vi "3D Experiment Final kinect.vi"() -> ()   [LabVIEW 2011]
uses:
  <vilib>/Platform/TimedLoop/XDataNode/timing_clust.ctl
  <vilib>/Platform/TimedLoop/XDataNode/nitl_modes.ctl
  <vilib>/Platform/TimedLoop/XDataNode/wakeup.ctl
  <vilib>/Utility/miscctls.llb/LV3DPointTypeDef.ctl
  <vilib>/Utility/miscctls.llb/LVRGBAColorTypeDef.ctl
  <vilib>/Utility/cursorutil.llb/Set Cursor (Cursor ID).vi
  <vilib>/Utility/inputDevices.llb/closeMouse.vi
  <vilib>/Utility/inputDevices.llb/mouseAcquire.vi
  <vilib>/Utility/file.llb/Write To Spreadsheet File (DBL).vi
  <vilib>/Utility/file.llb/Write To Spreadsheet File (I64).vi
  <vilib>/Platform/TimedLoop/XDataNode/XDataNode.xnode
  <vilib>/picture/3D Picture Control/NI_3D Picture Control.lvlib
  <vilib>/Platform/TimedLoop/XDataNode/XDNodeRunTimeDep.lvlib
  kinect-1-4/Kinect_API.lvlib
panel:
  in  "Far object filter 2":i32(slide)=26869 scale=0.0..4305.0
  out "click 2":bool
  out "stop":bool
  in  "Replace with?":i32=60000
  out "initial time 2":u32
  out "initial time":u32
  in  "stop":bool
  out "3D Picture":refnum<vi>(3d-picture)
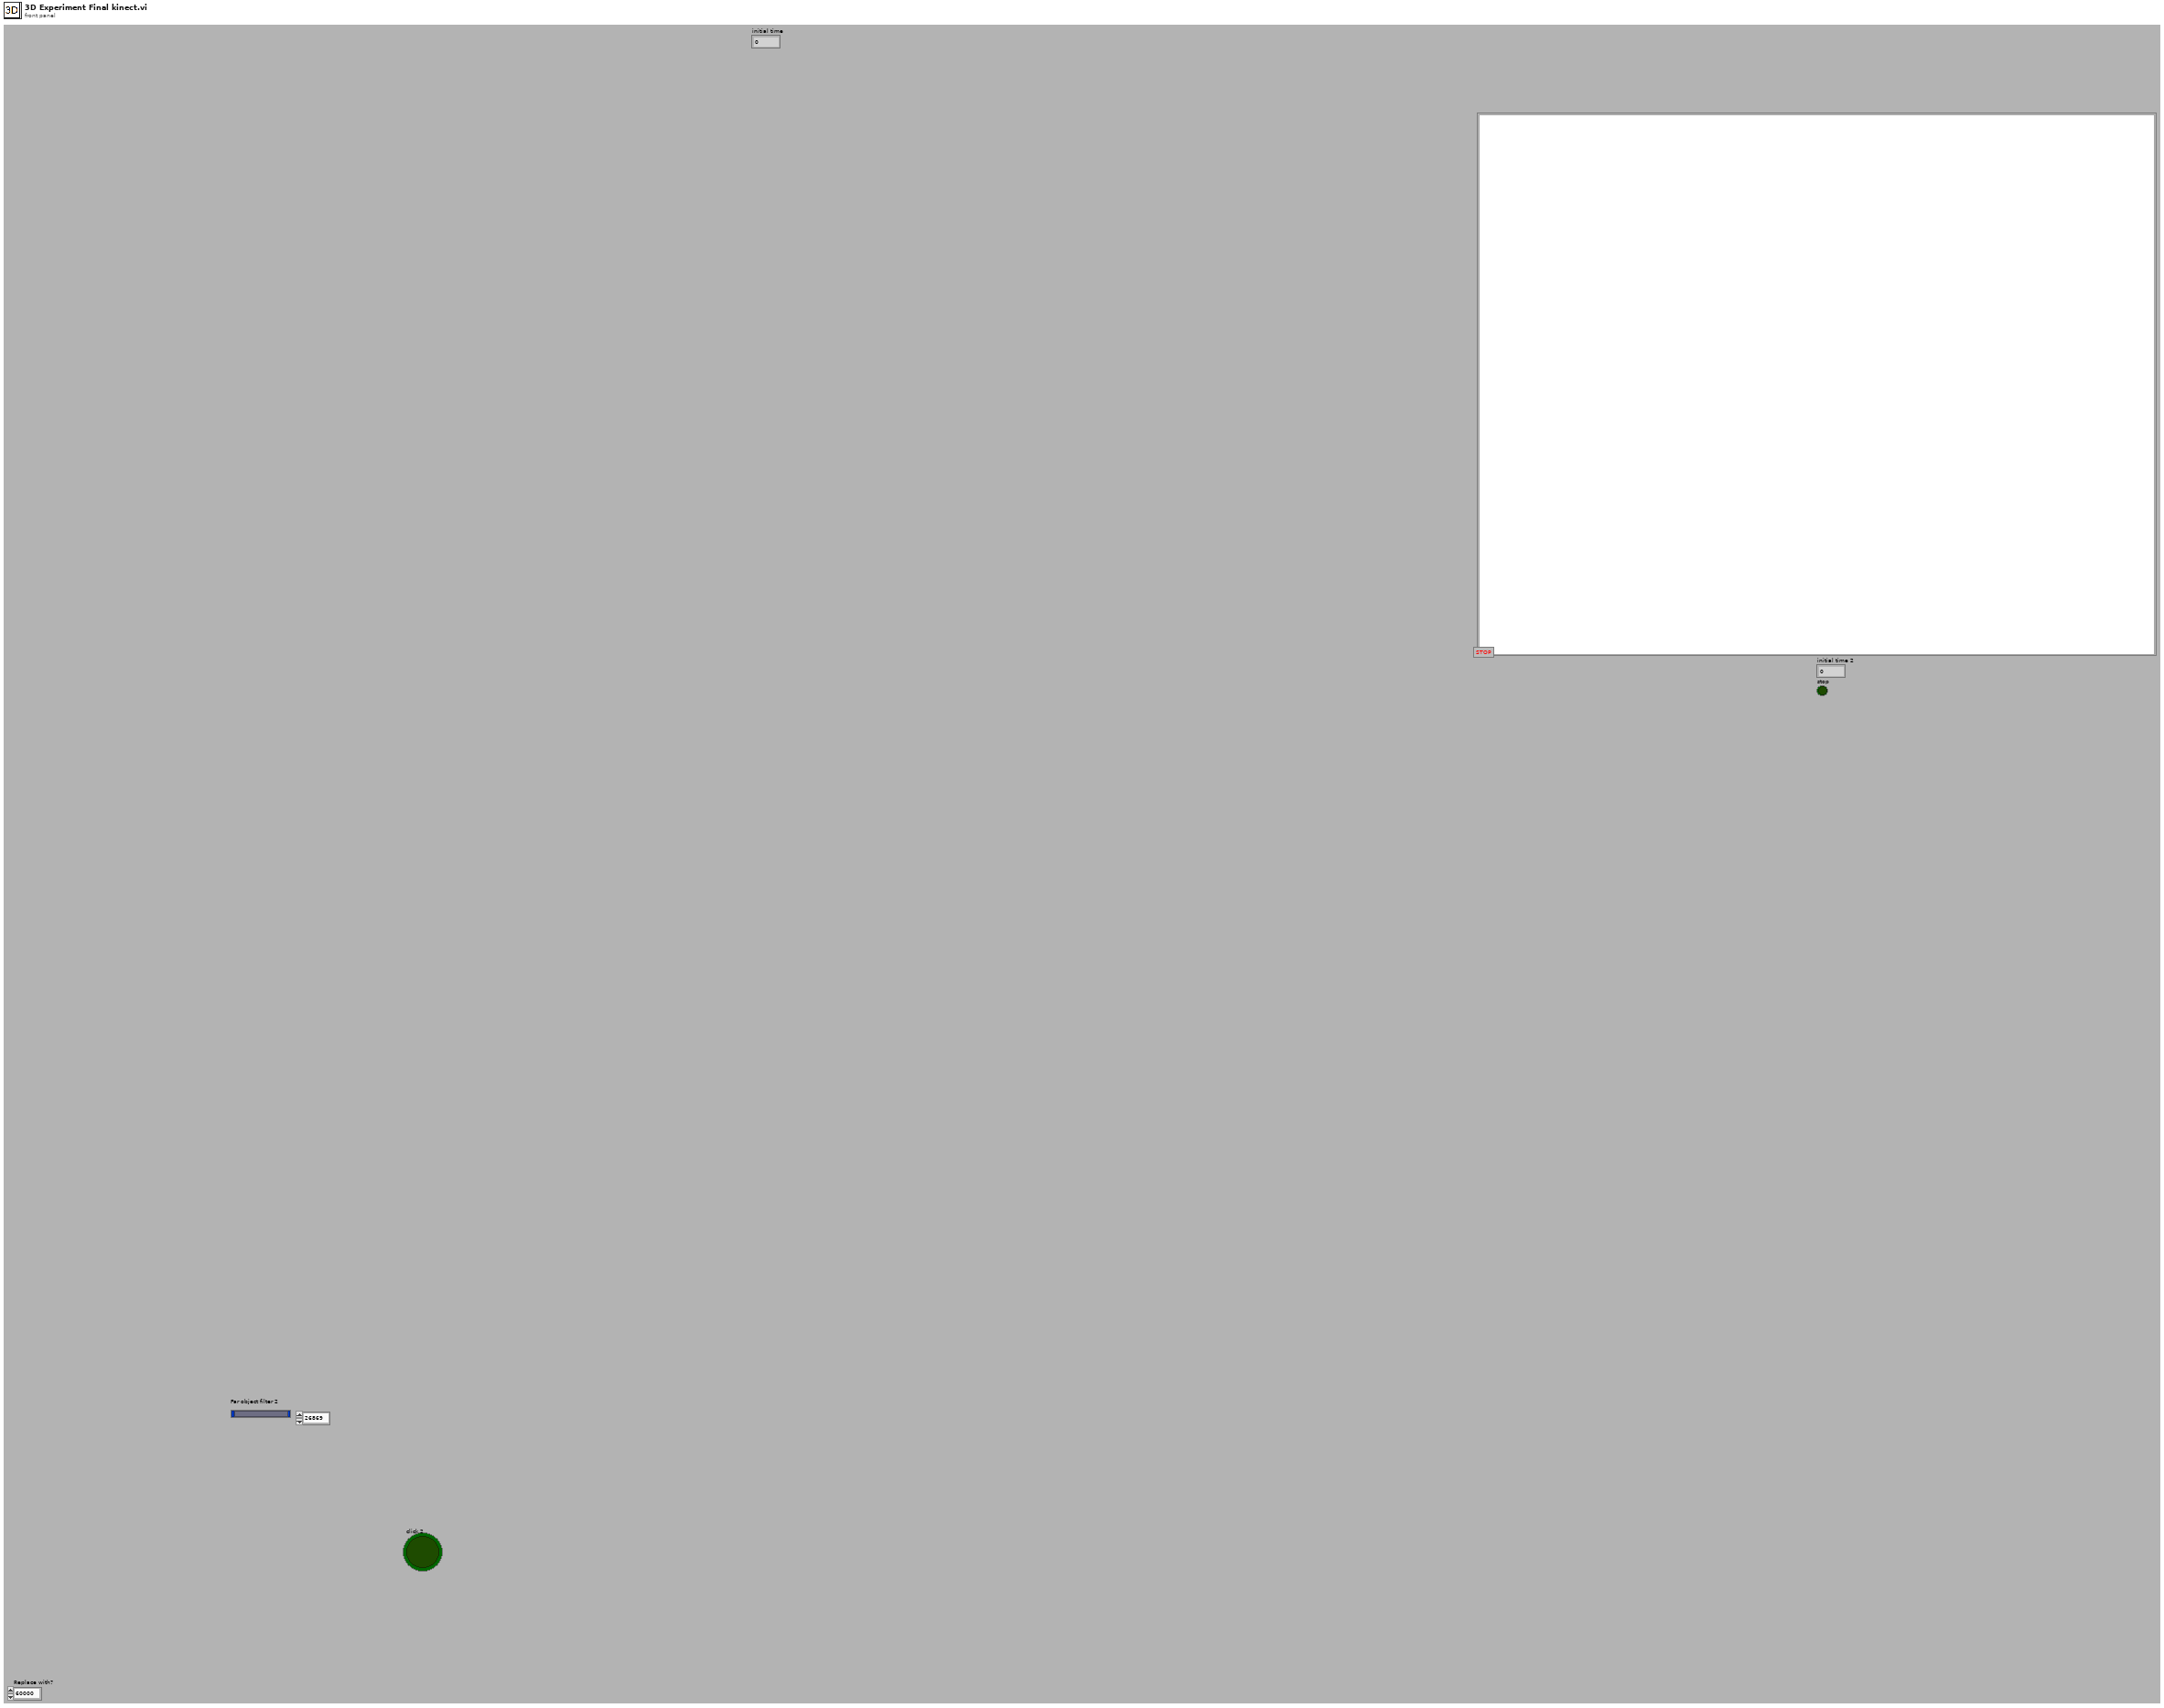
[diagram p1: front panel]
types:
  T1 = enum16{"open", "replace", "create", "open or create", "replace or create", "replace or create with confirmation"}
  T2 = typedef "LV3DPointTypeDef.ctl" = cluster{"X":sgl, "Y":sgl, "Z":sgl}
  T3 = enum16{"Inherit Value", "Points", "Wireframe", "Polygons"}
  T4 = enum16{"Inherit Value", "No Culling", "Cull Back Face", "Cull Front Face", "Cull Both Faces"}
  T5 = enum16{"Zero", "One", "Destination Color", "One Minus Destination Color", "Source Alpha", "One Minus Source Alpha", "Destination Alpha", "One Minus Destination Alpha", "Source Alpha Saturate"}
  T6 = enum16{"Zero", "One", "Source Color", "One Minus Source Color", "Source Alpha", "One Minus Source Alpha", "Destination Alpha", "One Minus Destination Alpha"}
  T7 = enum16{"Normal Bin", "Opaque Bin", "Transparent Bin"}
  T8 = typedef "XDNodeRunTimeDep.lvlib/timing_clust.ctl" = cluster{"Expected End [f-1]":u64, "Actual End [f-1]":u64, "Finished Late? [f-1]":bool, "Expected End [i-1]":u64, "Actual End [i-1]":u64, "Finished Late? [i-1]":bool, "Expected Start [i]":u64, "Actual Start [i]":u64, "Expected Start [f]":u64, "Actual Start [f]":u64, "Source Name":string, "Structure Name":string, "Period":i64, "Deadline":i64, "Offset":i64, "Start":i64, "Priority":i32, "Timeout":i32, "Mode":T9, "Wakeup Reason":T10, "Error":errorcluster, "Source Type":string, "Secondary Source Type":string, "Global End Time":u64, "Global Start Time":u64, "Frame Duration":u64, "Iteration Duration":u64, "Assigned CPU":i32, "I/O Scan Engine Mode":u32}
  T9 = typedef "XDNodeRunTimeDep.lvlib/nitl_modes.ctl" = enum32{"No Change", "Process missed periods, maintain original phase", "Discard missed periods, maintain original phase", "Process missed periods, ignore original phase", "Discard missed periods, ignore original phase"}
  T10 = typedef "XDNodeRunTimeDep.lvlib/wakeup.ctl" = enum32{"Normal", "Aborted", "Asynchronous wakeup", "Timing source error", "Timed loop error", "Timeout"}
  T11 = cluster{"Red":sgl, "Green":sgl, "Blue":sgl, "Alpha":sgl}
  T12 = typedef "LVRGBAColorTypeDef.ctl" = cluster{"Red":sgl, "Green":sgl, "Blue":sgl, "Alpha":sgl}
  T13 = typedef "LVAllMonitorsDisplayTypeDef.ctl" = cluster{"Bounds":cluster{"Left":i16, "Top":i16, "Right":i16, "Bottom":i16}, "Depth":i16}[]
  T14 = cluster{"Bounds":cluster{"Left":i16, "Top":i16, "Right":i16, "Bottom":i16}, "Depth":i16}
  T15 = cluster{"Left":i16, "Top":i16, "Right":i16, "Bottom":i16}
  T16 = cluster{"element":dbl, "Y_scaling":dbl, "element":dbl}
  T17 = cluster{"queue out":refnum<queue>, "queue out":refnum<queue>}
  T18 = cluster{"new reference":refnum<k24>, "DepthStream":refnum<k24>, "VideoStream":refnum<k24>, "Event Callback":refnum<k27>, "Event Callback":refnum<k27>}
  T19 = cluster{"button 1":bool, "button 2":bool, "button 3":bool, "button 4":bool}
  T20 = cluster{"\naverage Y":dbl, "\naverage X ":dbl, "average Z":dbl}
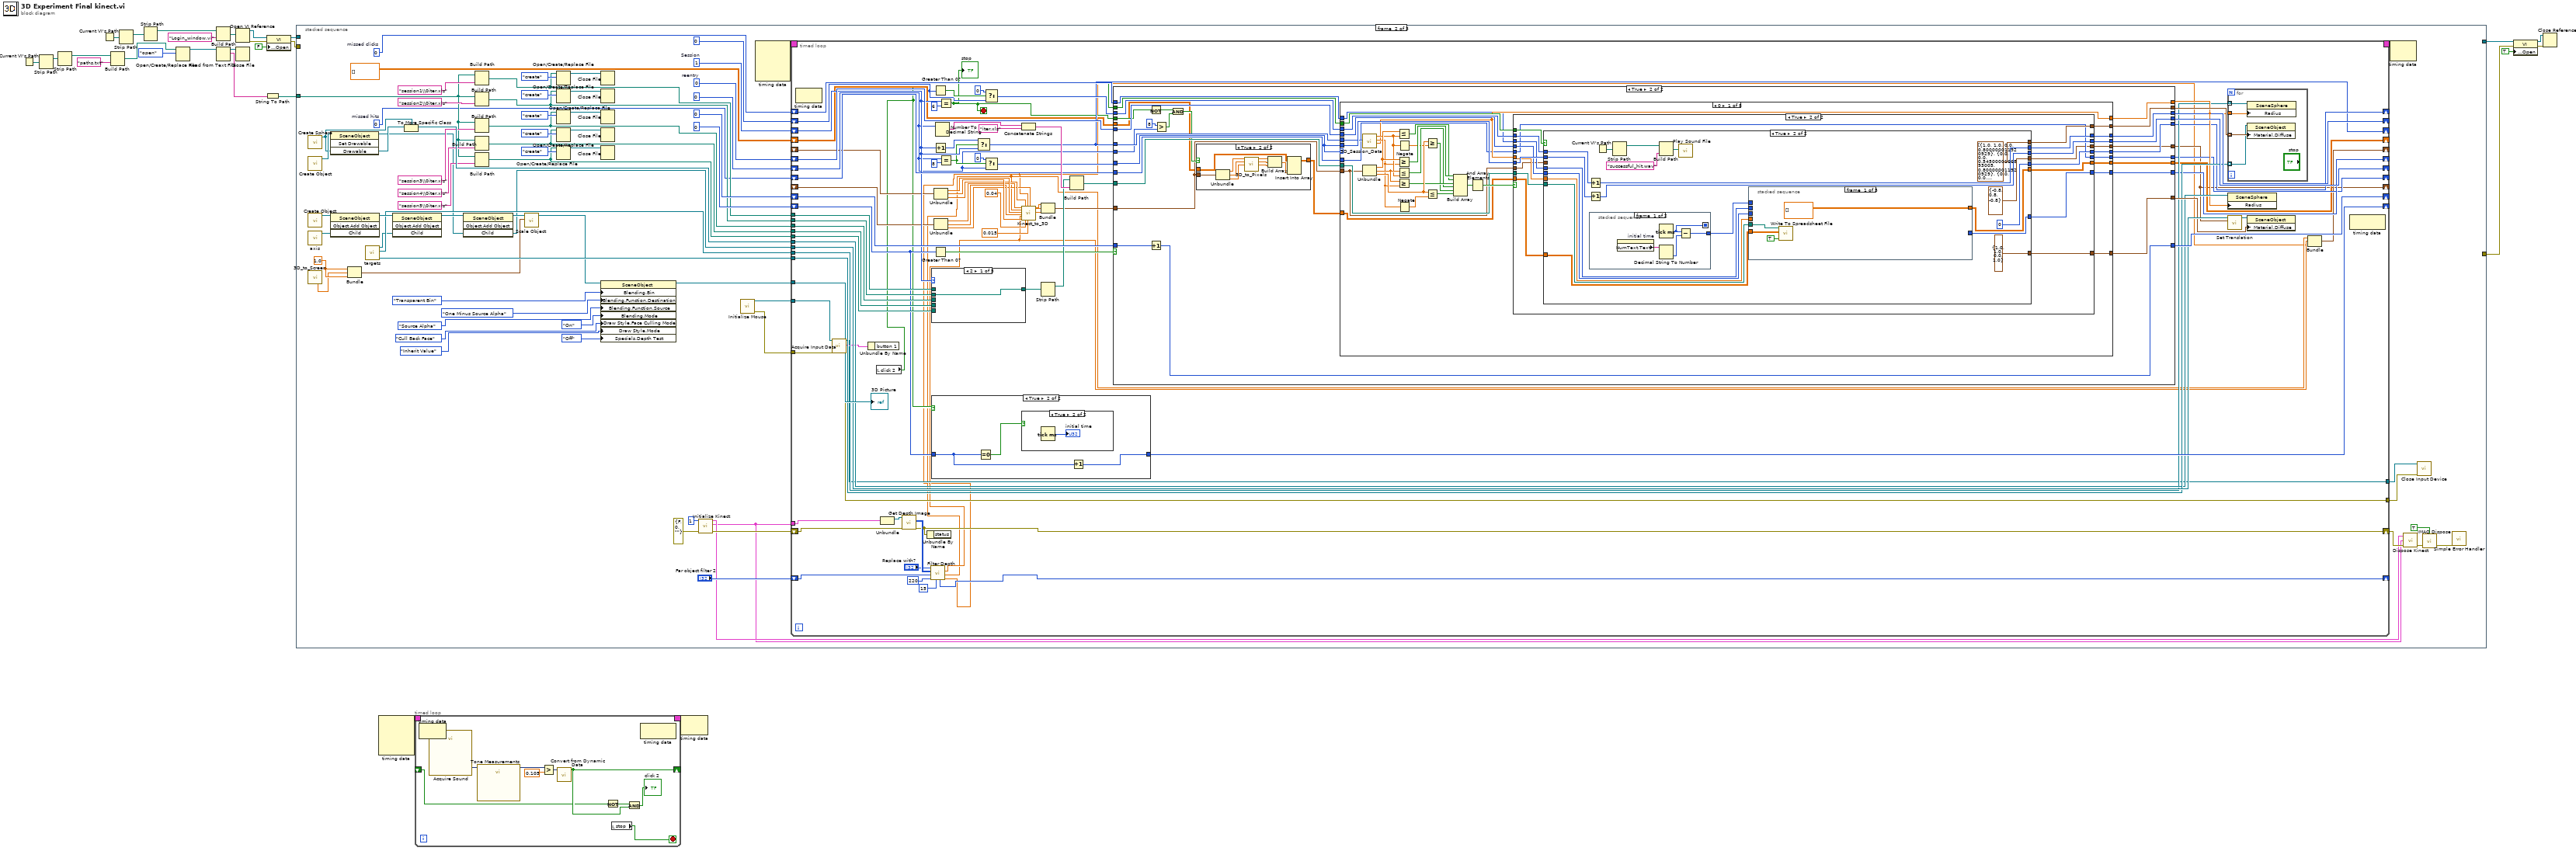
[diagram p0: block diagram]
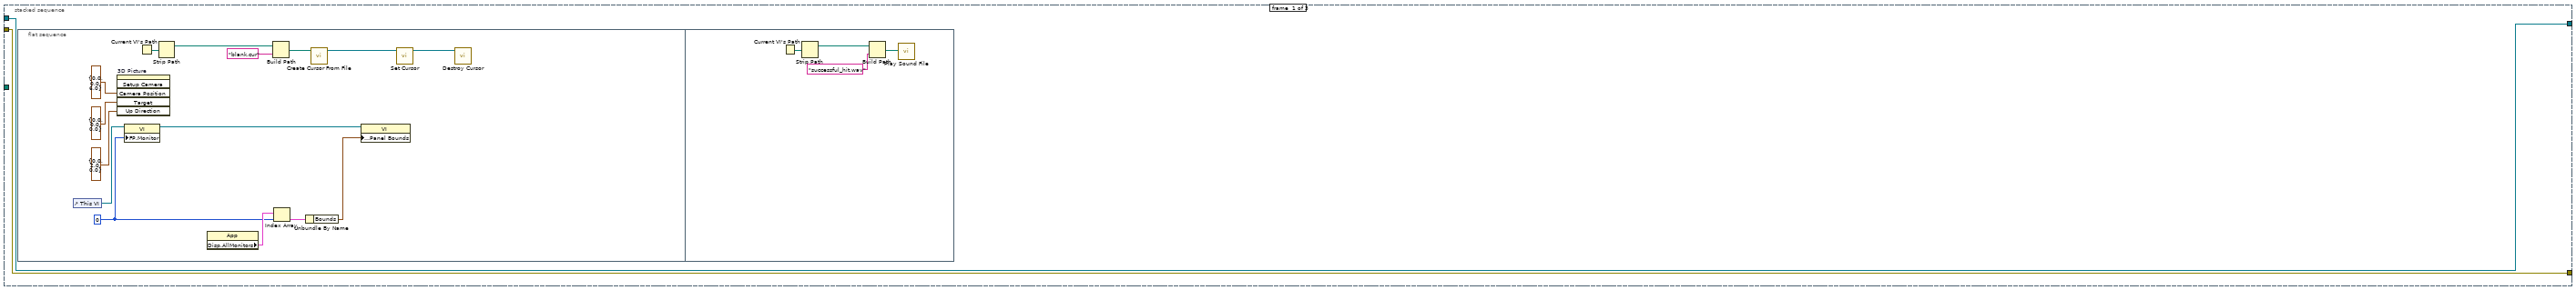
[diagram p2: hidden frame]
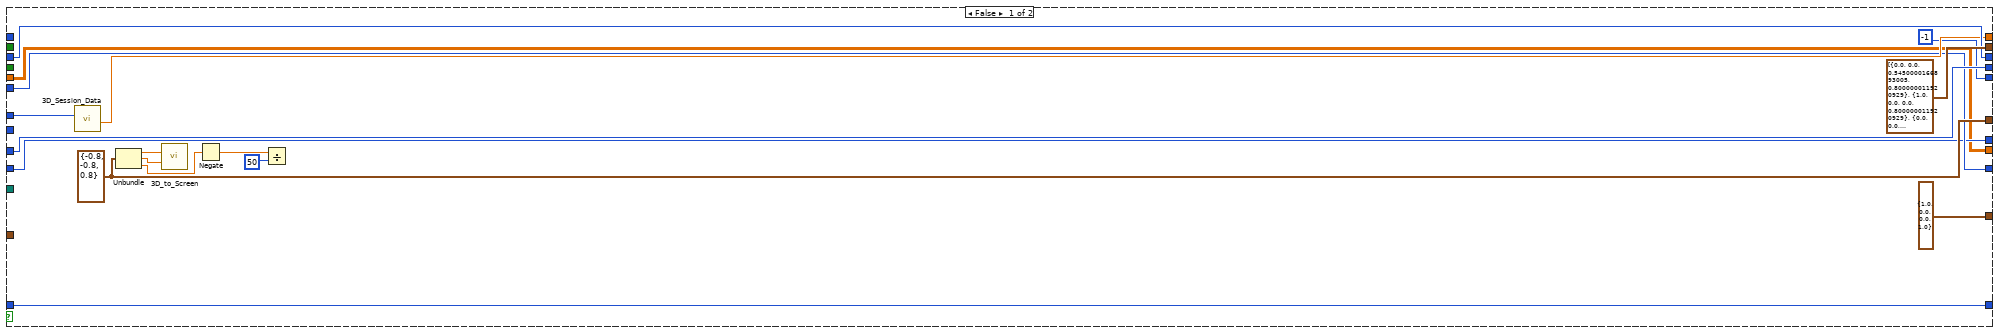
[diagram p7: hidden frame]
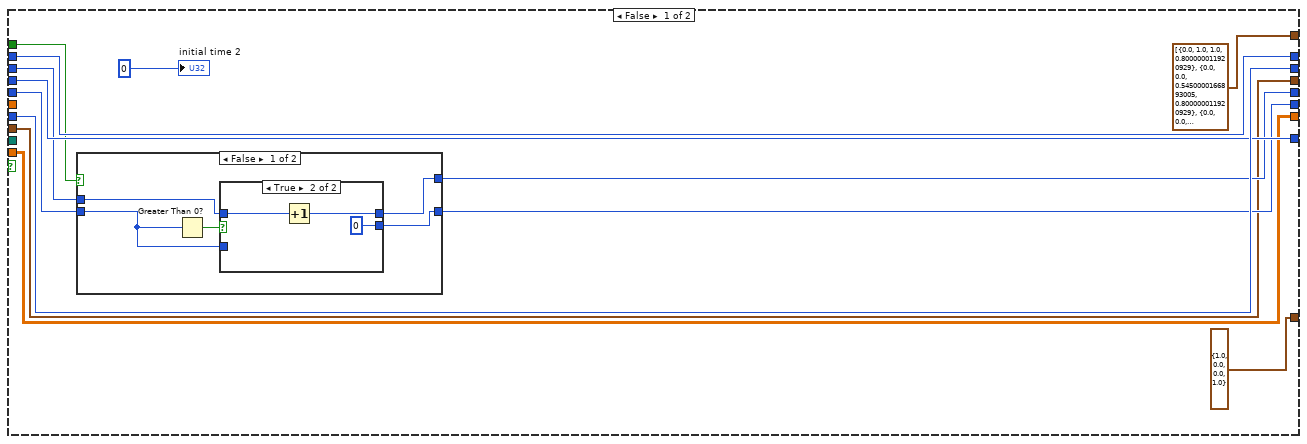
[diagram p9: hidden frame]
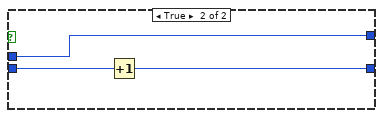
[diagram p11: hidden frame]
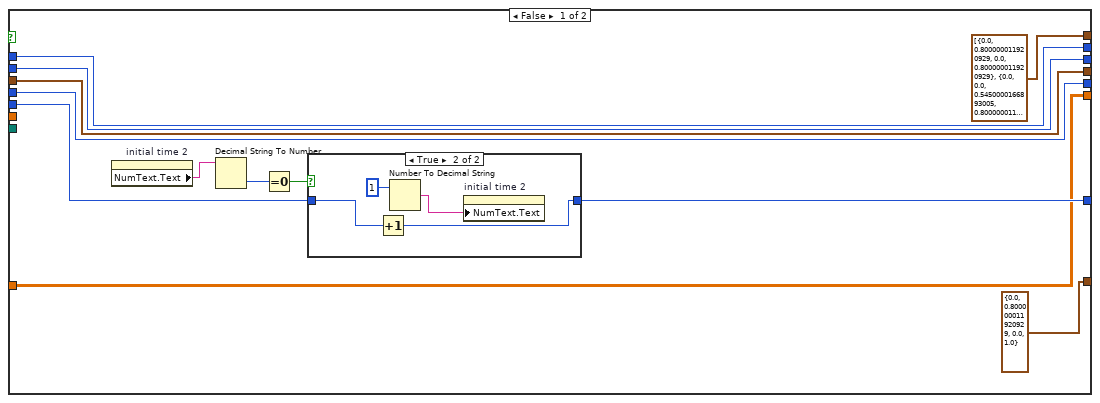
[diagram p12: hidden frame]
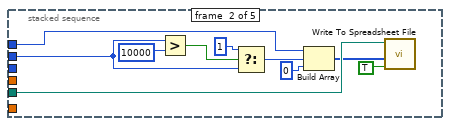
[diagram p14: hidden frame]
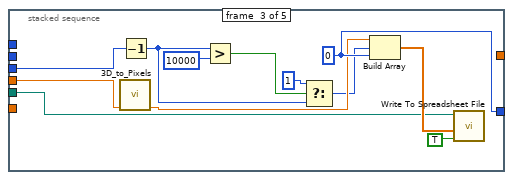
[diagram p15: hidden frame]
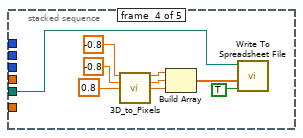
[diagram p16: hidden frame]
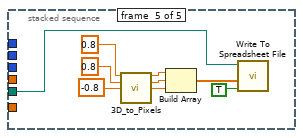
[diagram p17: hidden frame]
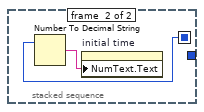
[diagram p18: hidden frame]
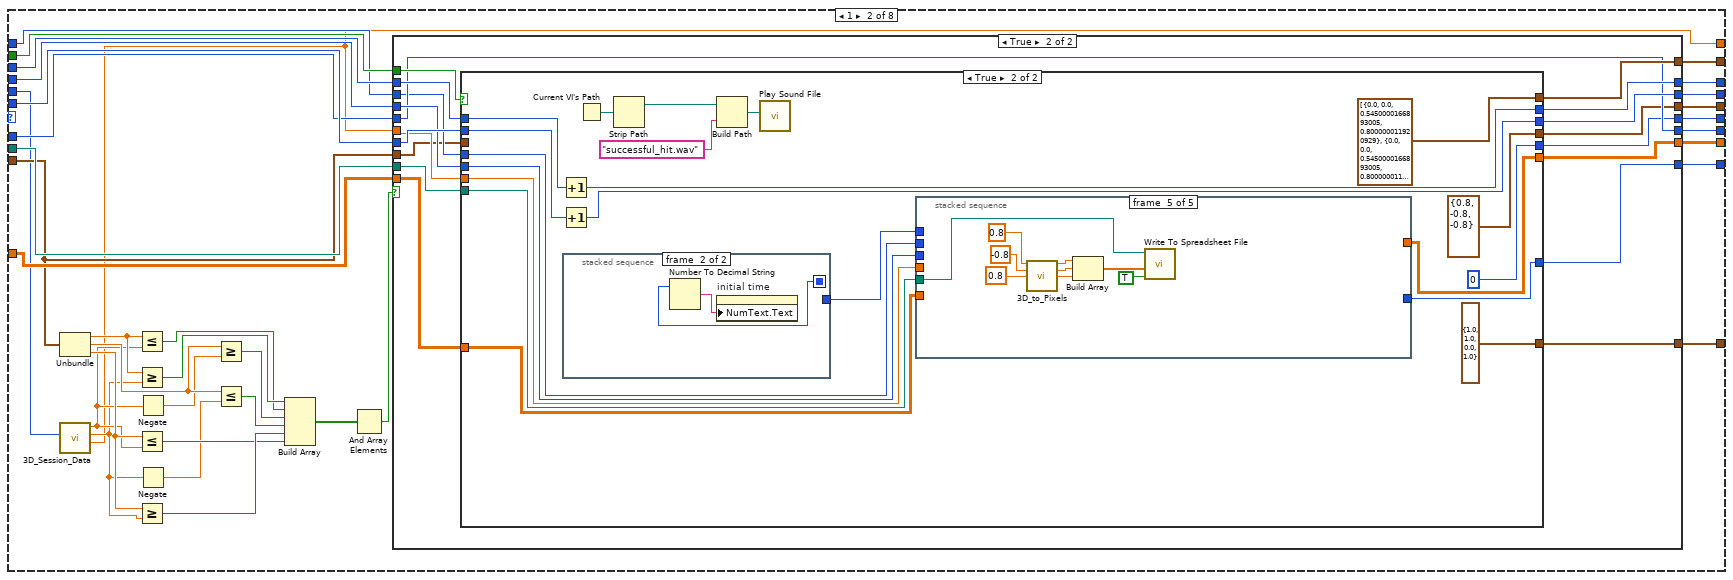
[diagram p19: hidden frame]
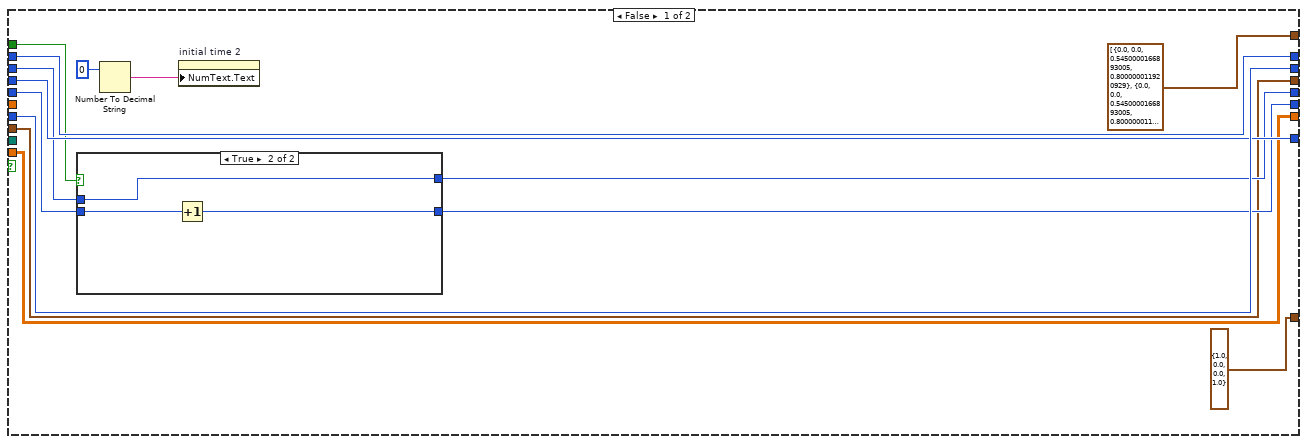
[diagram p20: hidden frame]
diagram:
  n1 = Current VI's Path() -> (path=w3:path)
  n2 = Strip Path(path=w3) -> (stripped path=w4:path)  [unwired: 1 out]
  n3 = Strip Path(path=w4) -> (stripped path=w21:path)  [unwired: 1 out]
  n4 = Current VI's Path() -> (path=w16:path)
  n5 = Build Path(base path=w21, name or relative path="paths.txt") -> (appended path=w24:path)
  n6 = Strip Path(path=w16) -> (stripped path=w13:path)  [unwired: 1 out]
  n7 = Strip Path(path=w13) -> (stripped path=w12:path)  [unwired: 1 out]
  n8 = Open/Create/Replace File(file path (use dialog)=w24, operation (0:open)=T1."open") -> (refnum out=w26:refnum<file>)  [unwired: 4 in, 2 out]
  n9 = Build Path(base path=w12, name or relative path="Login_window.vi") -> (appended path=w14:path)
  n10 = Read from Text File(file (use dialog)=w26) -> (refnum out=w27:refnum<file>, text=w25:string)  [unwired: 3 in, 2 out]
  n11 = Open VI Reference(vi path=w14) -> (vi reference=w19:refnum<vi>, error out=w18:errorcluster)  [unwired: 5 in]
  n12 = Close File(refnum=w27) -> ()  [unwired: 1 in, 2 out]
  n13 = String To Path(string=w25) -> (path=w20:path)
  n14 = property class="VI"(reference=w19, error in=w18, "Front Panel Window:Open"=FALSE) -> (reference out=w11:refnum<vi>, error out=w10:errorcluster)
  n15 = stacked-sequence {
    tunnel: w20 -> [_ w80 _]
    tunnel: w11 -> [w29 _ _]
    tunnel: w10 -> [w28 _ _]
    tunnel: [w29 _ _] -> w6
    tunnel: [w28 _ _] -> w5
    frame #0 {
      n16 = flat-sequence {
        frame #0 {
          w41 = u16 0 ("Front Panel Window:Monitor")
          n17 = control-ref of="This VI"() -> (w39:refnum<vi>)
          n18 = invoke on="3D Picture" class="SceneGraphDisp (strict)" method="Setup Camera"("Camera Position"=T2 {"X"=0.0, "Y"=0.0, "Z"=6.0}, "Target"=T2 {"X"=0.0, "Y"=0.0, "Z"=0.0}, "Up Direction"=T2 {"X"=0.0, "Y"=2.0, "Z"=0.0}) -> ()  [unwired: 3 in, 6 out]
          n19 = property class="VI"(reference=w39, "FP.Monitor"=w41) -> (reference out=w43:refnum<vi>)  [unwired: 1 in, 1 out]
          n20 = Current VI's Path() -> (path=w35:path)
          n21 = Strip Path(path=w35) -> (stripped path=w34:path)  [unwired: 1 out]
          n22 = property class="App"() -> ("Disp.AllMonitors"=w42:T13)  [unwired: 2 in, 2 out]
          n23 = Build Path(base path=w34, name or relative path="blank.cur") -> (appended path=w32:path)
          n24 = Index Array(array=w42, index=w41) -> (element=w40:T14)
          n25 = Unbundle By Name(w40) -> ("Bounds"=w44:T15)
          n26 = call <vilib>:"Create Cursor From File.vi"("cursor file"=w32) -> ("cursor ID"=w31:refnum<k1>)  [unwired: 9 in, 1 out]
          n27 = property class="VI"(reference=w43, "Front Panel Window:Panel Bounds"=w44) -> ()  [unwired: 1 in, 2 out]
          n28 = call-poly <vilib>:"Set Cursor.vi"("cursor ID"=w31) -> ("previous cursor ID"=w30:refnum<k1>)  [unwired: 9 in, 1 out]
          n29 = call <vilib>:"Destroy Cursor.vi"("cursor ID"=w30) -> ()  [unwired: 9 in, 1 out]
        }
        frame #1 {
          n30 = Current VI's Path() -> (path=w47:path)
          n31 = Strip Path(path=w47) -> (stripped path=w46:path)  [unwired: 1 out]
          n32 = Build Path(base path=w46, name or relative path="successful_hit.wav") -> (appended path=w48:path)
          n33 = call <vilib>:"Play Sound File.vi"("path"=w48) -> ()  [unwired: 9 in, 2 out]
        }
      }
    }
    frame #1 {
      w67 = 1.0 ("element")
      w68 = 0  # missed clicks
      w69 = 0  # missed hits
      w74 = 0  # reentry
      w109 = 1  # Session
      n34 = call <vilib>:"Create Sphere.vi"() -> ("New Sphere Refnum"=w107:refnum<vi>)  [unwired: 10 in, 1 out]
      n35 = call <vilib>:"Create Object.vi"() -> ("Scene:New Object"=w114:refnum<vi>)  [unwired: 10 in, 1 out]
      n36 = call <vilib>:"Create Object.vi"() -> ("Scene:New Object"=w113:refnum<vi>)  [unwired: 10 in, 1 out]
      n37 = call "axis.vi"() -> ("reference out"=w71:refnum<vi>)  [unwired: 11 in]
      n38 = call "3D_to_Screen.vi"() -> ("Y_scaling"=w64:dbl)  [unwired: 13 in, 2 out]
      n39 = invoke class="SceneObject" method="Object.Add Object"(reference=w113, "Child"=w71) -> (reference out=w112:refnum<vi>)  [unwired: 2 in, 3 out]
      n40 = invoke class="SceneObject" method="Set Drawable"(reference=w114, "Drawable"=w107) -> (reference out=w72:refnum<vi>, "Drawable"=w106:refnum<vi>)  [unwired: 2 in, 2 out]
      n41 = Bundle("element"=w67, "Y_scaling"=w64, "element"=w67) -> (w66:T16)  [unwired: 1 in]
      n42 = call "targets.vi"() -> ("objects"=w108:refnum<vi>[], "shperes"=w104:refnum<vi>[], "Scene:New Object"=w70:refnum<vi>)  [unwired: 8 in]
      n43 = invoke class="SceneObject" method="Object.Add Object"(reference=w112, "Child"=w70) -> (reference out=w111:refnum<vi>)  [unwired: 2 in, 3 out]
      n44 = To More Specific Class(target class=w107, reference=w106) -> (specific class reference=w105:refnum<vi>)  [unwired: 1 in, 1 out]
      n45 = invoke class="SceneObject" method="Object.Add Object"(reference=w111, "Child"=w72) -> (reference out=w110:refnum<vi>, "Child"=w73:refnum<vi>)  [unwired: 2 in, 2 out]
      n46 = Build Path(base path=w80, name or relative path="session1\\0iter.xls") -> (appended path=w75:path)
      n47 = Build Path(base path=w80, name or relative path="session2\\0iter.xls") -> (appended path=w76:path)
      n48 = Build Path(base path=w80, name or relative path="session3\\0iter.xls") -> (appended path=w78:path)
      n49 = Build Path(base path=w80, name or relative path="session4\\0iter.xls") -> (appended path=w77:path)
      n50 = Build Path(base path=w80, name or relative path="session5\\0iter.xls") -> (appended path=w79:path)
      n51 = call <vilib>:"Scale Object.vi"("Scale"=w66, "Scene.Object In"=w110) -> ("Scene.Object Out"=w65:refnum<vi>)  [unwired: 8 in, 1 out]
      n52 = Open/Create/Replace File(file path (use dialog)=w75, operation (0:open)=T1."create") -> (refnum out=w88:refnum<file>)  [unwired: 4 in, 2 out]
      n53 = Open/Create/Replace File(file path (use dialog)=w76, operation (0:open)=T1."create") -> (refnum out=w90:refnum<file>)  [unwired: 4 in, 2 out]
      n54 = Open/Create/Replace File(file path (use dialog)=w78, operation (0:open)=T1."create") -> (refnum out=w85:refnum<file>)  [unwired: 4 in, 2 out]
      n55 = Open/Create/Replace File(file path (use dialog)=w77, operation (0:open)=T1."create") -> (refnum out=w82:refnum<file>)  [unwired: 4 in, 2 out]
      n56 = Open/Create/Replace File(file path (use dialog)=w79, operation (0:open)=T1."create") -> (refnum out=w83:refnum<file>)  [unwired: 4 in, 2 out]
      n57 = Close File(refnum=w88) -> ()  [unwired: 1 in, 2 out]
      n58 = Close File(refnum=w90) -> ()  [unwired: 1 in, 2 out]
      n59 = Close File(refnum=w85) -> ()  [unwired: 1 in, 2 out]
      n60 = Close File(refnum=w82) -> ()  [unwired: 1 in, 2 out]
      n61 = Close File(refnum=w83) -> ()  [unwired: 1 in, 2 out]
      n62 = property class="SceneObject"(reference=w65, "Blending.Bin"=T7."Transparent Bin" ("Blending:Bin"), "Blending.Function.Destination"=T6."One Minus Source Alpha" ("Blending:Function:Destination"), "Blending.Function.Source"=T5."Source Alpha" ("Blending:Function:Source"), "Blending.Mode"=enum16{"Inherit Value", "Off", "On"}."On" ("Blending:Mode"), "Draw Style.Face Culling Mode"=T4."Cull Back Face" ("Draw Style:Face Culling Mode"), "Draw Style.Mode"=T3."Inherit Value" ("Draw Style:Mode"), "Specials.Depth Test"=enum16{"Inherit Value", "Off", "On"}."Off" ("Specials:Depth Test")) -> (reference out=w96:refnum<vi>)  [unwired: 1 in, 1 out]
      n63 = call "Initialize Kinect.vi"("error in (no error)"=errorcluster {"status"=FALSE, "code"=0, "source"=""}, "Buffer Size"=1) -> ("error out"=w55:errorcluster, "Queues Out"=w49:T17, "References"=w50:T18)  [unwired: 7 in]
      n64 = call <vilib>:"Initialize Mouse.vi"() -> ("error out"=w62:errorcluster, "device ID"=w60:refnum<k1>)  [unwired: 10 in]
      n65 = node-c288() -> (w120:T8)  [unwired: 4 in]
      n66 = timed-loop {
        shift-right: [w204] -> _
        shift-left: 0 ("y") -> [w175]
        shift-right: [w203] -> _
        shift-left: 0 ("y") -> [w161]
        shift-right: [w202] -> _
        shift-left: 0 ("y") -> [w166]
        timing: w120 -> [_]
        timing-out: [_] -> w119
        shift-right: [w160] -> _
        shift-left: w109 -> [w163]
        shift-right: [w198] -> _
        shift-left: 0 ("y") -> [w199]
        tunnel: w96 -> [w197]
        tunnel: w73 -> [w196]
        tunnel: w108 -> [w193]
        tunnel: w105 -> [w191]
        tunnel: w104 -> [w189]
        tunnel: w79 -> [w185]
        tunnel: w78 -> [w184]
        tunnel: w77 -> [w183]
        tunnel: w76 -> [w182]
        tunnel: w75 -> [w181]
        shift-right: [w176] -> _
        shift-left: w74 -> [w177]
        shift-right: [w171] -> _
        shift-left: w69 -> [w173]
        shift-right: [w170] -> _
        shift-left: w68 -> [w172]
        shift-right: [w158] -> _
        shift-left: dbl[][] [] -> [w155]
        shift-right: [w154] -> _
        shift-left: _ -> [w153]
        shift-right: [w148] -> _
        shift-left: _ -> [w147]
        tunnel: w62 -> [w141]
        tunnel: [w140] -> w61
        tunnel: w60 -> [w139]
        tunnel: [w138] -> w59
        shift-right: [w127] -> _
        shift-left: "Far object filter 2" -> [w128]
        shift-right: [w129] -> w51
        shift-left: w55 -> [w130]
        tunnel: w49 -> [w131]
        stop <- w143 stop-if-true
        n67 = node-c288() -> ()  [unwired: 1 in, 1 out]
        n68 = call-poly <vilib>:"Acquire Input Data.vi"("device ID"=w139, "error in (no error)"=w141) -> ("device ID"=w138:refnum<k1>, "button info"=w142:T19, "error out"=w140:errorcluster)  [unwired: 1 in, 14 out]
        n69 = Unbundle By Name(w142) -> ()  [unwired: 1 out]
        n70 = local read "click 2"() -> (w137:bool)
        n71 = Unbundle(w131) -> ("queue out"=w132:refnum<queue>)  [unwired: 1 out]
        n72 = call "Get Depth Image.vi"("error in (no error)"=w130, "queue in"=w132) -> ("error out"=w129:errorcluster, "Depth Image Pixels (U16)"=w134:u16[][])  [unwired: 6 in, 2 out]
        n73 = Unbundle By Name(w129) -> ()  [unwired: 1 out]
        n74 = call "Filter Depth.vi"("Wall-Threshold"=15, "Y-Threshold"=220, "Far object filter"=w128, "Depth Image Pixels (U16)"=w134, "Replace with?"="Replace with?") -> ("average Z"=w124:dbl, "average Y"=w125:dbl, "average X"=w126:dbl, "New far object filter"=w127:i32)  [unwired: 1 in, 2 out]
        n75 = case shown="2" w163 {
          tunnel: w185 -> [_ _ _ w208 _]
          tunnel: w183 -> [_ _ w207 _ _]
          tunnel: w184 -> [_ w206 _ _ _]
          tunnel: w182 -> [w205 _ _ _ _]
          tunnel: w181 -> [_ _ _ _ w209]
          tunnel: [w205 w206 w207 w208 w209] -> w178
          frame 2 {
          }
          frame 3 {
          }
          frame 4 {
          }
          frame 5 {
          }
          frame 1, Default {
          }
        }
        n76 = case shown="True" w137 {
          tunnel: w175 -> [w1606 w1607]
          tunnel: [w1606 w1609] -> w204
          frame False {
          }
          frame True {
            n77 = Equal To 0?(x=w1607) -> (x = 0?=w1608:bool)
            n78 = case shown="True" w1608 {
              frame False {
              }
              frame True {
                n79 = Tick Count (ms)() -> (millisecond timer value=→"initial time":u32)
              }
            }
            n80 = Increment(x=w1607) -> (x+1=w1609:i32)
          }
        }
        n81 = Greater Than 0?(x=w166) -> (x > 0?=w167:bool)
        n82 = Increment(x=w163) -> (x+1=w164:i32)
        n83 = Greater Than 0?(x=w175) -> (x > 0?=w174:bool)
        n84 = Unbundle(w153) -> ("average Y"=w152:dbl, "average X"=w151:dbl, "average Z"=w150:dbl)
        n85 = Unbundle(w147) -> ("X_3D"=w146:dbl, "Y_3D"=w145:dbl, "y"=w144:dbl)
        n86 = Number To Decimal String(number=w161) -> (decimal integer string=w186:string)  [unwired: 1 in]
        n87 = Equal?(x=w163, y=6) -> (x = y?=w143:bool)
        "stop" <- w143
        n88 = Equal?(x=w161, y=8) -> (x = y?=w162:bool)
        n89 = Select(t=w164, s=w162, f=w163) -> (s? t:f=w160:i32)
        n90 = Select(t=0 ("y"), s=w167, f=w166) -> (s? t:f=w168:i32)
        n91 = Select(t=0 ("y"), s=w162, f=w161) -> (s? t:f=w159:i32)
        n92 = Concatenate Strings(w186, "iter.xls" ("name or relative path")) -> (w187:string)
        n93 = call "Kinect_to_3D.vi"("previous_X_3D"=w146, "current_X_kinect"=w125, "previous_X_kinect"=w152, "previous_Y_3D"=w145, "current_Y_kinect"=w126, "previous_Y_kinect"=w151, "previous_Z_kinect"=w150, "X_Y_speed"=0.04, "current_Z_kinect"=w124, "Z_speed"=0.015, "previous_Z_3D"=w144) -> ("X_3D"=w121:dbl, "Y_3D"=w122:dbl, "Z_3D"=w123:dbl)  [unwired: 3 in, 3 out]
        n94 = Bundle("X_3D"=w121, "Y_3D"=w122, "Z_3D"=w123) -> (w149:cluster{"X_3D":dbl, "Y_3D":dbl, "Z_3D":dbl})  [unwired: 1 in]
        n95 = Strip Path(path=w178) -> (stripped path=w179:path)  [unwired: 1 out]
        n96 = Build Path(base path=w179, name or relative path=w187) -> (appended path=w180:path)
        n97 = case shown="True" w174 {
          tunnel: w149 -> [_ w236]
          tunnel: [w229 w243] -> w148
          tunnel: [T12[] [{"Red"=0.0, "Green"=0.0, "Blue"=0.545, "Alpha"=0.8}, {"Red"=1.0, "Green"=0.0, "Blue"=0.0, "Alpha"=0.8}, {"Red"=0.0, "Green"=0.0, "Blue"=0.545, "Alpha"=0.8}, {"Red"=0.0, "Green"=0.0, "Blue"=0.545, "Alpha"=0.8}, {"Red"=0.0, "Green"=0.0, "Blue"=0.545, "Alpha"=0.8}, {"Red"=0.0, "Green"=0.0, "Blue"=0.545, "Alpha"=0.8}, {"Red"=0.0, "Green"=0.0, "Blue"=0.545, "Alpha"=0.8}, {"Red"=0.0, "Green"=0.0, "Blue"=0.545, "Alpha"=0.8}] ("Array") w261] -> w192
          tunnel: w159 -> [w230 w242]
          tunnel: w137 -> [_ w259]
          tunnel: [T11 {"Red"=1.0, "Green"=0.0, "Blue"=0.0, "Alpha"=1.0} ("Color") w260] -> w195
          tunnel: [w230 w258] -> w203
          tunnel: w168 -> [w227 w257]
          tunnel: [w227 w256] -> w202
          tunnel: w160 -> [w225 w255]
          tunnel: w199 -> [w226 w254]
          tunnel: [w226 w253] -> w198
          tunnel: [w224 w252] -> w190
          tunnel: w180 -> [_ w248]
          tunnel: w177 -> [w223 w251]
          tunnel: [w223 w250] -> w176
          tunnel: w161 -> [_ w249]
          tunnel: w173 -> [w222 w247]
          tunnel: w172 -> [_ w246]
          tunnel: [-1 ("missed clicks") w244] -> w170
          tunnel: [w222 w245] -> w171
          tunnel: w143 -> [_ w240]
          tunnel: w155 -> [w216 w235]
          tunnel: [w216 w233] -> w158
          frame False {
            w229 = cluster{dbl, dbl, "y":dbl} {-0.8, -0.8, "y"=0.8}
            n98 = call "3D_Session_Data.vi"("Session"=w225) -> ("Radius"=w224:sgl)  [unwired: 8 in, 2 out]
            n99 = Unbundle(w229) -> (w221:dbl, w220:dbl, "y"=w217:dbl)
            n100 = call "3D_to_Screen.vi"("X_3D"=w221, "Y_3D"=w220) -> ()  [unwired: 11 in, 3 out]
            n101 = Negate(x=w217) -> (-x=w218:dbl)
            n102 = Divide(x=w218, y=50) -> ()  [unwired: 1 out]
          }
          frame True {
            n103 = Not(x=w240) -> (.not. x?=w239:bool)
            n104 = Increment(x=w254) -> (x+1=w253:i32)
            n105 = Greater?(x=8 ("y"), y=w249) -> (0:w238:bool)
            n106 = And(x=w239, y=w238) -> (x .and. y?=w237:bool)
            n107 = case shown="True" w237 {
              tunnel: w236 -> [_ w266]
              tunnel: w235 -> [w262 w265]
              tunnel: [w262 w263] -> w234
              frame False {
              }
              frame True {
                n108 = Unbundle(w266) -> ("X_3D"=w272:dbl, "Y_3D"=w271:dbl, "Z_3D"=w270:dbl)
                n109 = call "3D_to_Pixels.vi"("X_3D"=w272, "Y_3D"=w271, "Z_3D"=w270) -> ("X_pixels"=w269:dbl, "Y_pixels"=w268:dbl, "Z_pixels"=w267:dbl)  [unwired: 9 in, 1 out]
                n110 = Build Array(w269, w268, w267) -> (w264:dbl[])
                n111 = Insert Into Array(array=w265, new element=w264) -> (w263:dbl[][])  [unwired: 2 in]
              }
            }
            n112 = case shown="0" w242 {
              tunnel: [w307 w473 w640 w807 w972 w1139 w1306 w1473] -> w261
              tunnel: w236 -> [w276 w443 w608 w775 w940 w1107 w1273 w1441]
              tunnel: [w306 w472 w639 w806 w971 w1138 w1305 w1472] -> w260
              tunnel: w259 -> [w305 w471 w638 w805 w970 w1137 w1304 w1471]
              tunnel: w242 -> [w304 w470 w637 w804 w969 w1136 w1303 w1470]
              tunnel: [w303 w469 w636 w803 w968 w1135 w1302 w1469] -> w258
              tunnel: w257 -> [w291 w468 w635 w802 w967 w1134 w1301 w1468]
              tunnel: [w290 w467 w634 w801 w966 w1133 w1300 w1467] -> w256
              tunnel: w255 -> [w289 w442 w607 w774 w941 w1106 w1274 w1440]
              tunnel: [w283 w439 w606 w773 w942 w1105 w1272 w1439] -> w252
              tunnel: w248 -> [w284 w466 w633 w800 w965 w1132 w1299 w1466]
              tunnel: w251 -> [w281 w464 w631 w798 w963 w1130 w1297 w1465]
              tunnel: [w282 w465 w632 w799 w964 w1131 w1298 w1464] -> w250
              tunnel: w247 -> [w280 w463 w630 w797 w962 w1129 w1296 w1463]
              tunnel: w246 -> [w279 w462 w629 w796 w961 w1128 w1295 w1462]
              tunnel: [w278 w461 w628 w795 w960 w1127 w1294 w1461] -> w245
              tunnel: [w277 w460 w627 w794 w959 w1126 w1293 w1460] -> w244
              tunnel: [w275 w459 w626 w793 w958 w1125 w1292 w1459] -> w243
              tunnel: w234 -> [w274 w458 w625 w792 w957 w1124 w1291 w1458]
              tunnel: [w273 w457 w624 w791 w956 w1123 w1290 w1457] -> w233
              frame 0 {
                n113 = call "3D_Session_Data.vi"("Session"=w289) -> ("Radius"=w283:sgl, "min"=w287:dbl, "max"=w288:dbl)  [unwired: 8 in]
                n114 = Unbundle(w276) -> ("X_3D"=w302:dbl, "Y_3D"=w301:dbl, "Z_3D"=w300:dbl)
                n115 = Less Or Equal?(x=w302, y=w288) -> (x <= y?=w298:bool)
                n116 = Greater Or Equal?(x=w302, y=w287) -> (x >= y?=w299:bool)
                n117 = Less Or Equal?(x=w301, y=w288) -> (x <= y?=w296:bool)
                n118 = Greater Or Equal?(x=w301, y=w287) -> (x >= y?=w297:bool)
                n119 = Negate(x=w288) -> (-x=w286:dbl)
                n120 = Negate(x=w287) -> (-x=w285:dbl)
                n121 = Greater Or Equal?(x=w300, y=w286) -> (x >= y?=w295:bool)
                n122 = Less Or Equal?(x=w300, y=w285) -> (x <= y?=w294:bool)
                n123 = Build Array(w299, w298, w297, w296, w295, w294) -> (w293:bool[])
                n124 = And Array Elements(Boolean array=w293) -> (logical AND=w292:bool)
                n125 = case shown="True" w292 {
                  tunnel: [T12[] [{"Red"=0.0, "Green"=1.0, "Blue"=1.0, "Alpha"=0.8}, {"Red"=0.0, "Green"=0.0, "Blue"=0.545, "Alpha"=0.8}, {"Red"=0.0, "Green"=0.0, "Blue"=0.545, "Alpha"=0.8}, {"Red"=0.0, "Green"=0.0, "Blue"=0.545, "Alpha"=0.8}, {"Red"=0.0, "Green"=0.0, "Blue"=0.545, "Alpha"=0.8}, {"Red"=0.0, "Green"=0.0, "Blue"=0.545, "Alpha"=0.8}, {"Red"=0.0, "Green"=0.0, "Blue"=0.545, "Alpha"=0.8}, {"Red"=0.0, "Green"=0.0, "Blue"=0.545, "Alpha"=0.8}] ("Array") w351] -> w307
                  tunnel: [T11 {"Red"=1.0, "Green"=0.0, "Blue"=0.0, "Alpha"=1.0} ("Color") w350] -> w306
                  tunnel: w305 -> [w310 w349]
                  tunnel: w304 -> [w318 w348]
                  tunnel: [w318 w347] -> w303
                  tunnel: w291 -> [w317 w346]
                  tunnel: [w317 w345] -> w290
                  tunnel: w284 -> [_ w344]
                  tunnel: w283 -> [_ w343]
                  tunnel: [w316 w342] -> w282
                  tunnel: w281 -> [w316 w341]
                  tunnel: w280 -> [w314 w338]
                  tunnel: w279 -> [w313 w340]
                  tunnel: [w312 w338] -> w278
                  tunnel: [w311 w339] -> w277
                  tunnel: w276 -> [w309 w337]
                  tunnel: [w309 w336] -> w275
                  tunnel: w274 -> [w308 w335]
                  tunnel: [w308 w334] -> w273
                  frame False {
                    n126 = case shown="False" w310 {
                      tunnel: w314 -> [w322 w333]
                      tunnel: [w321 w332] -> w312
                      tunnel: w313 -> [w324 w331]
                      tunnel: [w323 w331] -> w311
                      frame False {
                        n127 = Greater Than 0?(x=w322) -> (x > 0?=w325:bool)
                        n128 = case shown="True" w325 {
                          tunnel: w324 -> [w327 w330]
                          tunnel: [w327 w329] -> w323
                          tunnel: w322 -> [w326 _]
                          tunnel: [w326 0 ("y")] -> w321
                          frame False {
                          }
                          frame True {
                            n129 = Increment(x=w330) -> (x+1=w329:i32)
                          }
                        }
                      }
                      frame True {
                        n130 = Increment(x=w333) -> (x+1=w332:i32)
                      }
                    }
                    "initial time 2" <- u32 0 ("initial time 2")
                  }
                  frame True {
                    n131 = case shown="True" w349 {
                      tunnel: [T12[] [{"Red"=0.0, "Green"=0.8, "Blue"=0.0, "Alpha"=0.8}, {"Red"=0.0, "Green"=0.0, "Blue"=0.545, "Alpha"=0.8}, {"Red"=0.0, "Green"=0.0, "Blue"=0.545, "Alpha"=0.8}, {"Red"=0.0, "Green"=0.0, "Blue"=0.545, "Alpha"=0.8}, {"Red"=0.0, "Green"=0.0, "Blue"=0.545, "Alpha"=0.8}, {"Red"=0.0, "Green"=0.0, "Blue"=0.545, "Alpha"=0.8}, {"Red"=0.0, "Green"=0.0, "Blue"=0.545, "Alpha"=0.8}, {"Red"=0.0, "Green"=0.0, "Blue"=0.545, "Alpha"=0.8}] ("Array") T12[] [{"Red"=1.0, "Green"=1.0, "Blue"=0.0, "Alpha"=0.8}, {"Red"=0.0, "Green"=0.0, "Blue"=0.545, "Alpha"=0.8}, {"Red"=0.0, "Green"=0.0, "Blue"=0.545, "Alpha"=0.8}, {"Red"=0.0, "Green"=0.0, "Blue"=0.545, "Alpha"=0.8}, {"Red"=0.0, "Green"=0.0, "Blue"=0.545, "Alpha"=0.8}, {"Red"=0.0, "Green"=0.0, "Blue"=0.545, "Alpha"=0.8}, {"Red"=0.0, "Green"=0.0, "Blue"=0.545, "Alpha"=0.8}, {"Red"=0.0, "Green"=0.0, "Blue"=0.545, "Alpha"=0.8}] ("Array")] -> w351
                      tunnel: [T11 {"Red"=0.0, "Green"=0.8, "Blue"=0.0, "Alpha"=1.0} ("Color") T11 {"Red"=1.0, "Green"=1.0, "Blue"=0.0, "Alpha"=1.0} ("Color")] -> w350
                      tunnel: w348 -> [w361 w386]
                      tunnel: [w361 w385] -> w347
                      tunnel: w346 -> [w360 w374]
                      tunnel: [w360 w373] -> w345
                      tunnel: w344 -> [_ w379]
                      tunnel: w343 -> [_ w378]
                      tunnel: [w355 w377] -> w342
                      tunnel: w341 -> [w356 w376]
                      tunnel: w340 -> [w354 w375]
                      tunnel: [w354 0 ("x")] -> w339
                      tunnel: w337 -> [w353 _]
                      tunnel: [w353 cluster{dbl, dbl, "y":dbl} {-0.8, 0.8, "y"=-0.8}] -> w336
                      tunnel: w335 -> [w352 w370]
                      tunnel: [w352 w369] -> w334
                      frame False {
                        n132 = property on="initial time 2" class="DigNum (strict)"() -> ("NumText.Text"=w358:string)  [unwired: 2 in, 2 out]
                        n133 = Decimal String To Number(string=w358) -> (number=w357:i32)  [unwired: 2 in, 1 out]
                        n134 = Equal To 0?(x=w357) -> (x = 0?=w359:bool)
                        n135 = case shown="True" w359 {
                          tunnel: w356 -> [w364 w368]
                          tunnel: [w364 w367] -> w355
                          frame False {
                          }
                          frame True {
                            n136 = Increment(x=w368) -> (x+1=w367:u32)
                            n137 = Number To Decimal String(number=1) -> (decimal integer string=w366:string)  [unwired: 1 in]
                            n138 = property on="initial time 2" class="DigNum (strict)"("NumText.Text"=w366) -> ()  [unwired: 2 in, 2 out]
                          }
                        }
                      }
                      frame True {
                        n139 = Increment(x=w374) -> (x+1=w373:i32)
                        n140 = Increment(x=w386) -> (x+1=w385:i32)
                        n141 = stacked-sequence {
                          seq-local: [w434 _] -> [_ w437]
                          tunnel: [w433 _] -> w380
                          frame #0 {
                            n142 = property on="initial time" class="DigNum (strict)"() -> ("NumText.Text"=w436:string)  [unwired: 2 in, 2 out]
                            n143 = Tick Count (ms)() -> (millisecond timer value=w434:u32)
                            n144 = Decimal String To Number(string=w436) -> (number=w435:i32)  [unwired: 2 in, 1 out]
                            n145 = Subtract(x=w434, y=w435) -> (x-y=w433:u32)
                          }
                          frame #1 {
                            n146 = Number To Decimal String(number=w437) -> (decimal integer string=w438:string)  [unwired: 1 in]
                            n147 = property on="initial time" class="DigNum (strict)"("NumText.Text"=w438) -> ()  [unwired: 2 in, 2 out]
                          }
                        }
                        n148 = Current VI's Path() -> (path=w383:path)
                        n149 = Strip Path(path=w383) -> (stripped path=w382:path)  [unwired: 1 out]
                        n150 = Build Path(base path=w382, name or relative path="successful_hit.wav") -> (appended path=w384:path)
                        n151 = call <vilib>:"Play Sound File.vi"("path"=w384) -> ()  [unwired: 9 in, 2 out]
                        n152 = stacked-sequence {
                          tunnel: w379 -> [w390 w401 w412 w422 w431]
                          tunnel: w380 -> [_ w399 _ _ _]
                          tunnel: w378 -> [_ _ w409 _ _]
                          tunnel: [_ _ w410 _ _] -> w377
                          tunnel: w376 -> [_ _ w411 _ _]
                          tunnel: w375 -> [_ w394 _ _ _]
                          tunnel: w370 -> [w391 _ _ _ _]
                          tunnel: [dbl[][] [] _ _ _ _] -> w369
                          frame #0 {
                            n153 = call-poly <vilib>:"Write To Spreadsheet File.vi"("append to file? (new file:F)"=TRUE, "2D data"=w391, "file path (dialog if empty)"=w390) -> ()  [unwired: 5 in, 1 out]
                          }
                          frame #1 {
                            n154 = Greater?(x=w394, y=u32 10000 ("element")) -> (0:w397:bool)
                            n155 = Select(t=1, s=w397, f=w394) -> (s? t:f=w393:i32)
                            n156 = Build Array(w399, w393, u32 0 ("element")) -> (w400:u32[])
                            n157 = call-poly <vilib>:"Write To Spreadsheet File.vi"("append to file? (new file:F)"=TRUE, "1D data"=w400, "file path (dialog if empty)"=w401) -> ()  [unwired: 5 in, 1 out]
                          }
                          frame #2 {
                            w410 = u32 0 ("element")
                            n158 = call "3D_to_Pixels.vi"("Distance_3D"=w409) -> ("Distance_pixels"=w408:dbl)  [unwired: 11 in, 3 out]
                            n159 = Decrement(x=w411) -> (x-1=w404:u32)
                            n160 = Greater?(x=w404, y=u32 10000 ("element")) -> (0:w407:bool)
                            n161 = Select(t=1, s=w407, f=w404) -> (s? t:f=w403:u32)
                            n162 = Build Array(w408, w403, w410) -> (w414:dbl[])
                            n163 = call-poly <vilib>:"Write To Spreadsheet File.vi"("append to file? (new file:F)"=TRUE, "1D data"=w414, "file path (dialog if empty)"=w412) -> ()  [unwired: 5 in, 1 out]
                          }
                          frame #3 {
                            n164 = call "3D_to_Pixels.vi"("X_3D"=-0.8 ("element"), "Y_3D"=-0.8 ("element"), "Z_3D"=0.8 ("element")) -> ("X_pixels"=w419:dbl, "Y_pixels"=w420:dbl, "Z_pixels"=w421:dbl)  [unwired: 9 in, 1 out]
                            n165 = Build Array(w419, w420, w421) -> (w418:dbl[])
                            n166 = call-poly <vilib>:"Write To Spreadsheet File.vi"("append to file? (new file:F)"=TRUE, "1D data"=w418, "file path (dialog if empty)"=w422) -> ()  [unwired: 5 in, 1 out]
                          }
                          frame #4 {
                            n167 = call "3D_to_Pixels.vi"("X_3D"=0.8 ("element"), "Y_3D"=0.8 ("element"), "Z_3D"=-0.8 ("element")) -> ("X_pixels"=w428:dbl, "Y_pixels"=w429:dbl, "Z_pixels"=w430:dbl)  [unwired: 9 in, 1 out]
                            n168 = Build Array(w428, w429, w430) -> (w427:dbl[])
                            n169 = call-poly <vilib>:"Write To Spreadsheet File.vi"("append to file? (new file:F)"=TRUE, "1D data"=w427, "file path (dialog if empty)"=w431) -> ()  [unwired: 5 in, 1 out]
                          }
                        }
                      }
                    }
                  }
                }
              }
              frame 1 {
                n170 = Unbundle(w443) -> ("X_3D"=w456:dbl, "Y_3D"=w455:dbl, "Z_3D"=w454:dbl)
                n171 = call "3D_Session_Data.vi"("Session"=w442) -> ("Radius"=w439:sgl, "min"=w440:dbl, "max"=w444:dbl)  [unwired: 8 in]
                n172 = Less Or Equal?(x=w456, y=w444) -> (x <= y?=w452:bool)
                n173 = Greater Or Equal?(x=w456, y=w440) -> (x >= y?=w453:bool)
                n174 = Less Or Equal?(x=w454, y=w444) -> (x <= y?=w448:bool)
                n175 = Greater Or Equal?(x=w454, y=w440) -> (x >= y?=w449:bool)
                n176 = Negate(x=w444) -> (-x=w446:dbl)
                n177 = Negate(x=w440) -> (-x=w445:dbl)
                n178 = Greater Or Equal?(x=w455, y=w446) -> (x >= y?=w451:bool)
                n179 = Less Or Equal?(x=w455, y=w445) -> (x <= y?=w450:bool)
                n180 = Build Array(w453, w452, w451, w450, w449, w448) -> (w447:bool[])
                n181 = And Array Elements(Boolean array=w447) -> (logical AND=w441:bool)
                n182 = case shown="True" w441 {
                  tunnel: [T12[] [{"Red"=0.0, "Green"=0.0, "Blue"=0.545, "Alpha"=0.8}, {"Red"=0.0, "Green"=0.0, "Blue"=0.545, "Alpha"=0.8}, {"Red"=0.0, "Green"=0.0, "Blue"=0.545, "Alpha"=0.8}, {"Red"=0.0, "Green"=0.0, "Blue"=0.545, "Alpha"=0.8}, {"Red"=0.0, "Green"=0.0, "Blue"=0.545, "Alpha"=0.8}, {"Red"=0.0, "Green"=0.0, "Blue"=0.545, "Alpha"=0.8}, {"Red"=0.0, "Green"=0.0, "Blue"=0.545, "Alpha"=0.8}, {"Red"=0.0, "Green"=1.0, "Blue"=1.0, "Alpha"=0.8}] ("Array") w518] -> w473
                  tunnel: [T11 {"Red"=1.0, "Green"=0.0, "Blue"=0.0, "Alpha"=1.0} ("Color") w517] -> w472
                  tunnel: w471 -> [w477 w516]
                  tunnel: w470 -> [w486 w515]
                  tunnel: [w486 w514] -> w469
                  tunnel: w468 -> [w485 w513]
                  tunnel: [w485 w512] -> w467
                  tunnel: w466 -> [_ w511]
                  tunnel: w439 -> [_ w510]
                  tunnel: [w484 w509] -> w465
                  tunnel: w464 -> [w484 w508]
                  tunnel: w463 -> [w481 w507]
                  tunnel: w462 -> [w480 w506]
                  tunnel: [w479 w507] -> w461
                  tunnel: [w478 w505] -> w460
                  tunnel: w443 -> [w476 w504]
                  tunnel: [w476 w503] -> w459
                  tunnel: w458 -> [w475 w502]
                  tunnel: [w475 w501] -> w457
                  frame False {
                    n183 = case shown="True" w477 {
                      tunnel: w481 -> [w489 w500]
                      tunnel: [w488 w499] -> w479
                      tunnel: w480 -> [w491 w498]
                      tunnel: [w490 w498] -> w478
                      frame False {
                        n184 = Greater Than 0?(x=w489) -> (x > 0?=w492:bool)
                        n185 = case shown="True" w492 {
                          tunnel: w491 -> [w494 w497]
                          tunnel: [w494 w496] -> w490
                          tunnel: w489 -> [w493 _]
                          tunnel: [w493 0 ("y")] -> w488
                          frame False {
                          }
                          frame True {
                            n186 = Increment(x=w497) -> (x+1=w496:i32)
                          }
                        }
                      }
                      frame True {
                        n187 = Increment(x=w500) -> (x+1=w499:i32)
                      }
                    }
                    n188 = Number To Decimal String(number=0) -> (decimal integer string=w483:string)  [unwired: 1 in]
                    n189 = property on="initial time 2" class="DigNum (strict)"("NumText.Text"=w483) -> ()  [unwired: 2 in, 2 out]
                  }
                  frame True {
                    n190 = case shown="True" w516 {
                      tunnel: [T12[] [{"Red"=0.0, "Green"=0.0, "Blue"=0.545, "Alpha"=0.8}, {"Red"=0.0, "Green"=0.0, "Blue"=0.545, "Alpha"=0.8}, {"Red"=0.0, "Green"=0.0, "Blue"=0.545, "Alpha"=0.8}, {"Red"=0.0, "Green"=0.0, "Blue"=0.545, "Alpha"=0.8}, {"Red"=0.0, "Green"=0.0, "Blue"=0.545, "Alpha"=0.8}, {"Red"=0.0, "Green"=0.0, "Blue"=0.545, "Alpha"=0.8}, {"Red"=0.0, "Green"=0.0, "Blue"=0.545, "Alpha"=0.8}, {"Red"=0.0, "Green"=0.8, "Blue"=0.0, "Alpha"=0.8}] ("Array") T12[] [{"Red"=0.0, "Green"=0.0, "Blue"=0.545, "Alpha"=0.8}, {"Red"=0.0, "Green"=0.0, "Blue"=0.545, "Alpha"=0.8}, {"Red"=0.0, "Green"=0.0, "Blue"=0.545, "Alpha"=0.8}, {"Red"=0.0, "Green"=0.0, "Blue"=0.545, "Alpha"=0.8}, {"Red"=0.0, "Green"=0.0, "Blue"=0.545, "Alpha"=0.8}, {"Red"=0.0, "Green"=0.0, "Blue"=0.545, "Alpha"=0.8}, {"Red"=0.0, "Green"=0.0, "Blue"=0.545, "Alpha"=0.8}, {"Red"=1.0, "Green"=1.0, "Blue"=0.0, "Alpha"=0.8}] ("Array")] -> w518
                      tunnel: [T11 {"Red"=0.0, "Green"=0.8, "Blue"=0.0, "Alpha"=1.0} ("Color") T11 {"Red"=1.0, "Green"=1.0, "Blue"=0.0, "Alpha"=1.0} ("Color")] -> w517
                      tunnel: w515 -> [w529 w554]
                      tunnel: [w529 w553] -> w514
                      tunnel: w513 -> [w528 w552]
                      tunnel: [w528 w551] -> w512
                      tunnel: w511 -> [_ w546]
                      tunnel: w510 -> [_ w544]
                      tunnel: [w524 w543] -> w509
                      tunnel: w508 -> [w523 w542]
                      tunnel: w506 -> [w522 w541]
                      tunnel: [w522 0 ("x")] -> w505
                      tunnel: w504 -> [w521 _]
                      tunnel: [w521 cluster{dbl, dbl, "y":dbl} {0.8, -0.8, "y"=-0.8}] -> w503
                      tunnel: w502 -> [w520 w538]
                      tunnel: [w520 w537] -> w501
                      frame False {
                        n191 = property on="initial time 2" class="DigNum (strict)"() -> ("NumText.Text"=w526:string)  [unwired: 2 in, 2 out]
                        n192 = Decimal String To Number(string=w526) -> (number=w525:i32)  [unwired: 2 in, 1 out]
                        n193 = Equal To 0?(x=w525) -> (x = 0?=w527:bool)
                        n194 = case shown="True" w527 {
                          tunnel: w523 -> [w531 w535]
                          tunnel: [w531 w534] -> w524
                          frame False {
                          }
                          frame True {
                            n195 = Increment(x=w535) -> (x+1=w534:u32)
                            n196 = Number To Decimal String(number=1) -> (decimal integer string=w533:string)  [unwired: 1 in]
                            n197 = property on="initial time 2" class="DigNum (strict)"("NumText.Text"=w533) -> ()  [unwired: 2 in, 2 out]
                          }
                        }
                      }
                      frame True {
                        n198 = Increment(x=w552) -> (x+1=w551:i32)
                        n199 = Increment(x=w554) -> (x+1=w553:i32)
                        n200 = stacked-sequence {
                          seq-local: [w601 _] -> [_ w604]
                          tunnel: [w600 _] -> w545
                          frame #0 {
                            n201 = property on="initial time" class="DigNum (strict)"() -> ("NumText.Text"=w603:string)  [unwired: 2 in, 2 out]
                            n202 = Tick Count (ms)() -> (millisecond timer value=w601:u32)
                            n203 = Decimal String To Number(string=w603) -> (number=w602:i32)  [unwired: 2 in, 1 out]
                            n204 = Subtract(x=w601, y=w602) -> (x-y=w600:u32)
                          }
                          frame #1 {
                            n205 = Number To Decimal String(number=w604) -> (decimal integer string=w605:string)  [unwired: 1 in]
                            n206 = property on="initial time" class="DigNum (strict)"("NumText.Text"=w605) -> ()  [unwired: 2 in, 2 out]
                          }
                        }
                        n207 = Current VI's Path() -> (path=w549:path)
                        n208 = Strip Path(path=w549) -> (stripped path=w548:path)  [unwired: 1 out]
                        n209 = Build Path(base path=w548, name or relative path="successful_hit.wav") -> (appended path=w550:path)
                        n210 = call <vilib>:"Play Sound File.vi"("path"=w550) -> ()  [unwired: 9 in, 2 out]
                        n211 = stacked-sequence {
                          tunnel: w546 -> [w557 w568 w579 w589 w598]
                          tunnel: w545 -> [_ w566 _ _ _]
                          tunnel: w544 -> [_ _ w576 _ _]
                          tunnel: [_ _ w577 _ _] -> w543
                          tunnel: w542 -> [_ _ w578 _ _]
                          tunnel: w541 -> [_ w561 _ _ _]
                          tunnel: w538 -> [w558 _ _ _ _]
                          tunnel: [dbl[][] [] _ _ _ _] -> w537
                          frame #0 {
                            n212 = call-poly <vilib>:"Write To Spreadsheet File.vi"("append to file? (new file:F)"=TRUE, "2D data"=w558, "file path (dialog if empty)"=w557) -> ()  [unwired: 5 in, 1 out]
                          }
                          frame #1 {
                            n213 = Greater?(x=w561, y=u32 10000 ("element")) -> (0:w564:bool)
                            n214 = Select(t=1, s=w564, f=w561) -> (s? t:f=w560:i32)
                            n215 = Build Array(w566, w560, u32 0 ("element")) -> (w567:u32[])
                            n216 = call-poly <vilib>:"Write To Spreadsheet File.vi"("append to file? (new file:F)"=TRUE, "1D data"=w567, "file path (dialog if empty)"=w568) -> ()  [unwired: 5 in, 1 out]
                          }
                          frame #2 {
                            w577 = u32 0 ("element")
                            n217 = call "3D_to_Pixels.vi"("Distance_3D"=w576) -> ("Distance_pixels"=w575:dbl)  [unwired: 11 in, 3 out]
                            n218 = Decrement(x=w578) -> (x-1=w571:u32)
                            n219 = Greater?(x=w571, y=u32 10000 ("element")) -> (0:w574:bool)
                            n220 = Select(t=1, s=w574, f=w571) -> (s? t:f=w570:u32)
                            n221 = Build Array(w575, w570, w577) -> (w581:dbl[])
                            n222 = call-poly <vilib>:"Write To Spreadsheet File.vi"("append to file? (new file:F)"=TRUE, "1D data"=w581, "file path (dialog if empty)"=w579) -> ()  [unwired: 5 in, 1 out]
                          }
                          frame #3 {
                            n223 = call "3D_to_Pixels.vi"("X_3D"=-0.8 ("element"), "Y_3D"=0.8 ("element"), "Z_3D"=-0.8 ("element")) -> ("X_pixels"=w586:dbl, "Y_pixels"=w587:dbl, "Z_pixels"=w588:dbl)  [unwired: 9 in, 1 out]
                            n224 = Build Array(w586, w587, w588) -> (w585:dbl[])
                            n225 = call-poly <vilib>:"Write To Spreadsheet File.vi"("append to file? (new file:F)"=TRUE, "1D data"=w585, "file path (dialog if empty)"=w589) -> ()  [unwired: 5 in, 1 out]
                          }
                          frame #4 {
                            n226 = call "3D_to_Pixels.vi"("X_3D"=0.8 ("element"), "Y_3D"=-0.8 ("element"), "Z_3D"=0.8 ("element")) -> ("X_pixels"=w595:dbl, "Y_pixels"=w596:dbl, "Z_pixels"=w597:dbl)  [unwired: 9 in, 1 out]
                            n227 = Build Array(w595, w596, w597) -> (w594:dbl[])
                            n228 = call-poly <vilib>:"Write To Spreadsheet File.vi"("append to file? (new file:F)"=TRUE, "1D data"=w594, "file path (dialog if empty)"=w598) -> ()  [unwired: 5 in, 1 out]
                          }
                        }
                      }
                    }
                  }
                }
              }
              frame 2 {
                n229 = Unbundle(w608) -> ("X_3D"=w623:dbl, "Y_3D"=w622:dbl, "Z_3D"=w621:dbl)
                n230 = call "3D_Session_Data.vi"("Session"=w607) -> ("Radius"=w606:sgl, "min"=w611:dbl, "max"=w610:dbl)  [unwired: 8 in]
                n231 = Less Or Equal?(x=w622, y=w610) -> (x <= y?=w617:bool)
                n232 = Greater Or Equal?(x=w622, y=w611) -> (x >= y?=w618:bool)
                n233 = Less Or Equal?(x=w621, y=w610) -> (x <= y?=w615:bool)
                n234 = Greater Or Equal?(x=w621, y=w611) -> (x >= y?=w616:bool)
                n235 = Negate(x=w610) -> (-x=w613:dbl)
                n236 = Negate(x=w611) -> (-x=w612:dbl)
                n237 = Greater Or Equal?(x=w623, y=w613) -> (x >= y?=w620:bool)
                n238 = Less Or Equal?(x=w623, y=w612) -> (x <= y?=w619:bool)
                n239 = Build Array(w620, w619, w618, w617, w616, w615) -> (w614:bool[])
                n240 = And Array Elements(Boolean array=w614) -> (logical AND=w609:bool)
                n241 = case shown="True" w609 {
                  tunnel: [T12[] [{"Red"=0.0, "Green"=0.0, "Blue"=0.545, "Alpha"=0.8}, {"Red"=0.0, "Green"=0.0, "Blue"=0.545, "Alpha"=0.8}, {"Red"=0.0, "Green"=0.0, "Blue"=0.545, "Alpha"=0.8}, {"Red"=0.0, "Green"=0.0, "Blue"=0.545, "Alpha"=0.8}, {"Red"=0.0, "Green"=1.0, "Blue"=1.0, "Alpha"=0.8}, {"Red"=0.0, "Green"=0.0, "Blue"=0.545, "Alpha"=0.8}, {"Red"=0.0, "Green"=0.0, "Blue"=0.545, "Alpha"=0.8}, {"Red"=0.0, "Green"=0.0, "Blue"=0.545, "Alpha"=0.8}] ("Array") w685] -> w640
                  tunnel: [T11 {"Red"=1.0, "Green"=0.0, "Blue"=0.0, "Alpha"=1.0} ("Color") w684] -> w639
                  tunnel: w638 -> [w648 w683]
                  tunnel: w637 -> [w653 w682]
                  tunnel: [w653 w681] -> w636
                  tunnel: w635 -> [w652 w680]
                  tunnel: [w652 w679] -> w634
                  tunnel: w633 -> [_ w678]
                  tunnel: w606 -> [_ w677]
                  tunnel: [w651 w676] -> w632
                  tunnel: w631 -> [w651 w675]
                  tunnel: w630 -> [w647 w674]
                  tunnel: w629 -> [w646 w673]
                  tunnel: [w645 w674] -> w628
                  tunnel: [w644 w672] -> w627
                  tunnel: w608 -> [w643 w671]
                  tunnel: [w643 w670] -> w626
                  tunnel: w625 -> [w642 w669]
                  tunnel: [w642 w668] -> w624
                  frame False {
                    n242 = case shown="False" w648 {
                      tunnel: w647 -> [w656 w667]
                      tunnel: [w655 w666] -> w645
                      tunnel: w646 -> [w658 w665]
                      tunnel: [w657 w665] -> w644
                      frame False {
                        n243 = Greater Than 0?(x=w656) -> (x > 0?=w659:bool)
                        n244 = case shown="True" w659 {
                          tunnel: w658 -> [w661 w664]
                          tunnel: [w661 w663] -> w657
                          tunnel: w656 -> [w660 _]
                          tunnel: [w660 0 ("y")] -> w655
                          frame False {
                          }
                          frame True {
                            n245 = Increment(x=w664) -> (x+1=w663:i32)
                          }
                        }
                      }
                      frame True {
                        n246 = Increment(x=w667) -> (x+1=w666:i32)
                      }
                    }
                    n247 = Number To Decimal String(number=0) -> (decimal integer string=w650:string)  [unwired: 1 in]
                    n248 = property on="initial time 2" class="DigNum (strict)"("NumText.Text"=w650) -> ()  [unwired: 2 in, 2 out]
                  }
                  frame True {
                    n249 = case shown="False" w683 {
                      tunnel: [T12[] [{"Red"=0.0, "Green"=0.0, "Blue"=0.545, "Alpha"=0.8}, {"Red"=0.0, "Green"=0.0, "Blue"=0.545, "Alpha"=0.8}, {"Red"=0.0, "Green"=0.0, "Blue"=0.545, "Alpha"=0.8}, {"Red"=0.0, "Green"=0.0, "Blue"=0.545, "Alpha"=0.8}, {"Red"=0.0, "Green"=0.8, "Blue"=0.0, "Alpha"=0.8}, {"Red"=0.0, "Green"=0.0, "Blue"=0.545, "Alpha"=0.8}, {"Red"=0.0, "Green"=0.0, "Blue"=0.545, "Alpha"=0.8}, {"Red"=0.0, "Green"=0.0, "Blue"=0.545, "Alpha"=0.8}] ("Array") T12[] [{"Red"=0.0, "Green"=0.0, "Blue"=0.545, "Alpha"=0.8}, {"Red"=0.0, "Green"=0.0, "Blue"=0.545, "Alpha"=0.8}, {"Red"=0.0, "Green"=0.0, "Blue"=0.545, "Alpha"=0.8}, {"Red"=0.0, "Green"=0.0, "Blue"=0.545, "Alpha"=0.8}, {"Red"=1.0, "Green"=1.0, "Blue"=0.0, "Alpha"=0.8}, {"Red"=0.0, "Green"=0.0, "Blue"=0.545, "Alpha"=0.8}, {"Red"=0.0, "Green"=0.0, "Blue"=0.545, "Alpha"=0.8}, {"Red"=0.0, "Green"=0.0, "Blue"=0.545, "Alpha"=0.8}] ("Array")] -> w685
                      tunnel: [T11 {"Red"=0.0, "Green"=0.8, "Blue"=0.0, "Alpha"=1.0} ("Color") T11 {"Red"=1.0, "Green"=1.0, "Blue"=0.0, "Alpha"=1.0} ("Color")] -> w684
                      tunnel: w682 -> [w696 w721]
                      tunnel: [w696 w720] -> w681
                      tunnel: w680 -> [w695 w719]
                      tunnel: [w695 w718] -> w679
                      tunnel: w678 -> [_ w712]
                      tunnel: w677 -> [_ w711]
                      tunnel: [w690 w710] -> w676
                      tunnel: w675 -> [w691 w709]
                      tunnel: w673 -> [w689 w708]
                      tunnel: [w689 0 ("x")] -> w672
                      tunnel: w671 -> [w688 _]
                      tunnel: [w688 cluster{dbl, dbl, "y":dbl} {0.8, 0.8, "y"=0.8}] -> w670
                      tunnel: w669 -> [w687 w705]
                      tunnel: [w687 w704] -> w668
                      frame False {
                        n250 = property on="initial time 2" class="DigNum (strict)"() -> ("NumText.Text"=w693:string)  [unwired: 2 in, 2 out]
                        n251 = Decimal String To Number(string=w693) -> (number=w692:i32)  [unwired: 2 in, 1 out]
                        n252 = Equal To 0?(x=w692) -> (x = 0?=w694:bool)
                        n253 = case shown="True" w694 {
                          tunnel: w691 -> [w698 w702]
                          tunnel: [w698 w701] -> w690
                          frame False {
                          }
                          frame True {
                            n254 = Increment(x=w702) -> (x+1=w701:u32)
                            n255 = Number To Decimal String(number=1) -> (decimal integer string=w700:string)  [unwired: 1 in]
                            n256 = property on="initial time 2" class="DigNum (strict)"("NumText.Text"=w700) -> ()  [unwired: 2 in, 2 out]
                          }
                        }
                      }
                      frame True {
                        n257 = Increment(x=w719) -> (x+1=w718:i32)
                        n258 = Increment(x=w721) -> (x+1=w720:i32)
                        n259 = stacked-sequence {
                          seq-local: [w768 _] -> [_ w771]
                          tunnel: [w767 _] -> w713
                          frame #0 {
                            n260 = property on="initial time" class="DigNum (strict)"() -> ("NumText.Text"=w770:string)  [unwired: 2 in, 2 out]
                            n261 = Tick Count (ms)() -> (millisecond timer value=w768:u32)
                            n262 = Decimal String To Number(string=w770) -> (number=w769:i32)  [unwired: 2 in, 1 out]
                            n263 = Subtract(x=w768, y=w769) -> (x-y=w767:u32)
                          }
                          frame #1 {
                            n264 = Number To Decimal String(number=w771) -> (decimal integer string=w772:string)  [unwired: 1 in]
                            n265 = property on="initial time" class="DigNum (strict)"("NumText.Text"=w772) -> ()  [unwired: 2 in, 2 out]
                          }
                        }
                        n266 = Current VI's Path() -> (path=w716:path)
                        n267 = Strip Path(path=w716) -> (stripped path=w715:path)  [unwired: 1 out]
                        n268 = Build Path(base path=w715, name or relative path="successful_hit.wav") -> (appended path=w717:path)
                        n269 = call <vilib>:"Play Sound File.vi"("path"=w717) -> ()  [unwired: 9 in, 2 out]
                        n270 = stacked-sequence {
                          tunnel: w712 -> [w724 w735 w746 w756 w765]
                          tunnel: w713 -> [_ w733 _ _ _]
                          tunnel: w711 -> [_ _ w743 _ _]
                          tunnel: [_ _ w744 _ _] -> w710
                          tunnel: w709 -> [_ _ w745 _ _]
                          tunnel: w708 -> [_ w728 _ _ _]
                          tunnel: w705 -> [w725 _ _ _ _]
                          tunnel: [dbl[][] [] _ _ _ _] -> w704
                          frame #0 {
                            n271 = call-poly <vilib>:"Write To Spreadsheet File.vi"("append to file? (new file:F)"=TRUE, "2D data"=w725, "file path (dialog if empty)"=w724) -> ()  [unwired: 5 in, 1 out]
                          }
                          frame #1 {
                            n272 = Greater?(x=w728, y=u32 10000 ("element")) -> (0:w731:bool)
                            n273 = Select(t=1, s=w731, f=w728) -> (s? t:f=w727:i32)
                            n274 = Build Array(w733, w727, u32 0 ("element")) -> (w734:u32[])
                            n275 = call-poly <vilib>:"Write To Spreadsheet File.vi"("append to file? (new file:F)"=TRUE, "1D data"=w734, "file path (dialog if empty)"=w735) -> ()  [unwired: 5 in, 1 out]
                          }
                          frame #2 {
                            w744 = u32 0 ("element")
                            n276 = call "3D_to_Pixels.vi"("Distance_3D"=w743) -> ("Distance_pixels"=w742:dbl)  [unwired: 11 in, 3 out]
                            n277 = Decrement(x=w745) -> (x-1=w738:u32)
                            n278 = Greater?(x=w738, y=u32 10000 ("element")) -> (0:w741:bool)
                            n279 = Select(t=1, s=w741, f=w738) -> (s? t:f=w737:u32)
                            n280 = Build Array(w742, w737, w744) -> (w747:dbl[])
                            n281 = call-poly <vilib>:"Write To Spreadsheet File.vi"("append to file? (new file:F)"=TRUE, "1D data"=w747, "file path (dialog if empty)"=w746) -> ()  [unwired: 5 in, 1 out]
                          }
                          frame #3 {
                            n282 = call "3D_to_Pixels.vi"("X_3D"=0.8 ("element"), "Y_3D"=-0.8 ("element"), "Z_3D"=-0.8 ("element")) -> ("X_pixels"=w753:dbl, "Y_pixels"=w754:dbl, "Z_pixels"=w755:dbl)  [unwired: 9 in, 1 out]
                            n283 = Build Array(w753, w754, w755) -> (w752:dbl[])
                            n284 = call-poly <vilib>:"Write To Spreadsheet File.vi"("append to file? (new file:F)"=TRUE, "1D data"=w752, "file path (dialog if empty)"=w756) -> ()  [unwired: 5 in, 1 out]
                          }
                          frame #4 {
                            n285 = call "3D_to_Pixels.vi"("X_3D"=-0.8 ("element"), "Y_3D"=0.8 ("element"), "Z_3D"=0.8 ("element")) -> ("X_pixels"=w762:dbl, "Y_pixels"=w763:dbl, "Z_pixels"=w764:dbl)  [unwired: 9 in, 1 out]
                            n286 = Build Array(w762, w763, w764) -> (w761:dbl[])
                            n287 = call-poly <vilib>:"Write To Spreadsheet File.vi"("append to file? (new file:F)"=TRUE, "1D data"=w761, "file path (dialog if empty)"=w765) -> ()  [unwired: 5 in, 1 out]
                          }
                        }
                      }
                    }
                  }
                }
              }
              frame 3 {
                n288 = call "3D_Session_Data.vi"("Session"=w774) -> ("Radius"=w773:sgl, "min"=w780:dbl, "max"=w777:dbl)  [unwired: 8 in]
                n289 = Unbundle(w775) -> ("X_3D"=w790:dbl, "Y_3D"=w789:dbl, "Z_3D"=w788:dbl)
                n290 = Negate(x=w777) -> (-x=w779:dbl)
                n291 = Negate(x=w780) -> (-x=w778:dbl)
                n292 = Greater Or Equal?(x=w790, y=w779) -> (x >= y?=w787:bool)
                n293 = Greater Or Equal?(x=w789, y=w779) -> (x >= y?=w785:bool)
                n294 = Greater Or Equal?(x=w788, y=w779) -> (x >= y?=w783:bool)
                n295 = Less Or Equal?(x=w790, y=w778) -> (x <= y?=w786:bool)
                n296 = Less Or Equal?(x=w789, y=w778) -> (x <= y?=w784:bool)
                n297 = Less Or Equal?(x=w788, y=w778) -> (x <= y?=w782:bool)
                n298 = Build Array(w787, w786, w785, w784, w783, w782) -> (w781:bool[])
                n299 = And Array Elements(Boolean array=w781) -> (logical AND=w776:bool)
                n300 = case shown="True" w776 {
                  tunnel: [T12[] [{"Red"=0.0, "Green"=0.0, "Blue"=0.545, "Alpha"=0.8}, {"Red"=0.0, "Green"=0.0, "Blue"=0.545, "Alpha"=0.8}, {"Red"=0.0, "Green"=0.0, "Blue"=0.545, "Alpha"=0.8}, {"Red"=0.0, "Green"=1.0, "Blue"=1.0, "Alpha"=0.8}, {"Red"=0.0, "Green"=0.0, "Blue"=0.545, "Alpha"=0.8}, {"Red"=0.0, "Green"=0.0, "Blue"=0.545, "Alpha"=0.8}, {"Red"=0.0, "Green"=0.0, "Blue"=0.545, "Alpha"=0.8}, {"Red"=0.0, "Green"=0.0, "Blue"=0.545, "Alpha"=0.8}] ("Array") w852] -> w807
                  tunnel: [T11 {"Red"=1.0, "Green"=0.0, "Blue"=0.0, "Alpha"=1.0} ("Color") w851] -> w806
                  tunnel: w805 -> [w811 w850]
                  tunnel: w804 -> [w820 w849]
                  tunnel: [w820 w848] -> w803
                  tunnel: w802 -> [w819 w847]
                  tunnel: [w819 w846] -> w801
                  tunnel: w800 -> [_ w845]
                  tunnel: w773 -> [_ w844]
                  tunnel: [w818 w843] -> w799
                  tunnel: w798 -> [w818 w842]
                  tunnel: w797 -> [w815 w841]
                  tunnel: w796 -> [w814 w840]
                  tunnel: [w813 w841] -> w795
                  tunnel: [w812 w839] -> w794
                  tunnel: w775 -> [w810 w838]
                  tunnel: [w810 w837] -> w793
                  tunnel: w792 -> [w809 w836]
                  tunnel: [w809 w835] -> w791
                  frame False {
                    n301 = case shown="False" w811 {
                      tunnel: w815 -> [w823 w834]
                      tunnel: [w822 w833] -> w813
                      tunnel: w814 -> [w825 w832]
                      tunnel: [w824 w832] -> w812
                      frame False {
                        n302 = Greater Than 0?(x=w823) -> (x > 0?=w826:bool)
                        n303 = case shown="True" w826 {
                          tunnel: w825 -> [w828 w831]
                          tunnel: [w828 w830] -> w824
                          tunnel: w823 -> [w827 _]
                          tunnel: [w827 0 ("y")] -> w822
                          frame False {
                          }
                          frame True {
                            n304 = Increment(x=w831) -> (x+1=w830:i32)
                          }
                        }
                      }
                      frame True {
                        n305 = Increment(x=w834) -> (x+1=w833:i32)
                      }
                    }
                    n306 = Number To Decimal String(number=0) -> (decimal integer string=w817:string)  [unwired: 1 in]
                    n307 = property on="initial time 2" class="DigNum (strict)"("NumText.Text"=w817) -> ()  [unwired: 2 in, 2 out]
                  }
                  frame True {
                    n308 = case shown="True" w850 {
                      tunnel: [T12[] [{"Red"=0.0, "Green"=0.0, "Blue"=0.545, "Alpha"=0.8}, {"Red"=0.0, "Green"=0.0, "Blue"=0.545, "Alpha"=0.8}, {"Red"=0.0, "Green"=0.0, "Blue"=0.545, "Alpha"=0.8}, {"Red"=0.0, "Green"=0.8, "Blue"=0.0, "Alpha"=0.8}, {"Red"=0.0, "Green"=0.0, "Blue"=0.545, "Alpha"=0.8}, {"Red"=0.0, "Green"=0.0, "Blue"=0.545, "Alpha"=0.8}, {"Red"=0.0, "Green"=0.0, "Blue"=0.545, "Alpha"=0.8}, {"Red"=0.0, "Green"=0.0, "Blue"=0.545, "Alpha"=0.8}] ("Array") T12[] [{"Red"=0.0, "Green"=0.0, "Blue"=0.545, "Alpha"=0.8}, {"Red"=0.0, "Green"=0.0, "Blue"=0.545, "Alpha"=0.8}, {"Red"=0.0, "Green"=0.0, "Blue"=0.545, "Alpha"=0.8}, {"Red"=1.0, "Green"=1.0, "Blue"=0.0, "Alpha"=0.8}, {"Red"=0.0, "Green"=0.0, "Blue"=0.545, "Alpha"=0.8}, {"Red"=0.0, "Green"=0.0, "Blue"=0.545, "Alpha"=0.8}, {"Red"=0.0, "Green"=0.0, "Blue"=0.545, "Alpha"=0.8}, {"Red"=0.0, "Green"=0.0, "Blue"=0.545, "Alpha"=0.8}] ("Array")] -> w852
                      tunnel: [T11 {"Red"=0.0, "Green"=0.8, "Blue"=0.0, "Alpha"=1.0} ("Color") T11 {"Red"=1.0, "Green"=1.0, "Blue"=0.0, "Alpha"=1.0} ("Color")] -> w851
                      tunnel: w849 -> [w863 w888]
                      tunnel: [w863 w887] -> w848
                      tunnel: w847 -> [w862 w886]
                      tunnel: [w862 w885] -> w846
                      tunnel: w845 -> [_ w879]
                      tunnel: w844 -> [_ w878]
                      tunnel: [w857 w877] -> w843
                      tunnel: w842 -> [w858 w876]
                      tunnel: w840 -> [w856 w875]
                      tunnel: [w856 0 ("x")] -> w839
                      tunnel: w838 -> [w855 _]
                      tunnel: [w855 cluster{dbl, dbl, "y":dbl} {-0.8, -0.8, "y"=-0.8}] -> w837
                      tunnel: w836 -> [w854 w872]
                      tunnel: [w854 w871] -> w835
                      frame False {
                        n309 = property on="initial time 2" class="DigNum (strict)"() -> ("NumText.Text"=w860:string)  [unwired: 2 in, 2 out]
                        n310 = Decimal String To Number(string=w860) -> (number=w859:i32)  [unwired: 2 in, 1 out]
                        n311 = Equal To 0?(x=w859) -> (x = 0?=w861:bool)
                        n312 = case shown="False" w861 {
                          tunnel: w858 -> [w865 w869]
                          tunnel: [w865 w868] -> w857
                          frame False {
                          }
                          frame True {
                            n313 = Increment(x=w869) -> (x+1=w868:u32)
                            n314 = Number To Decimal String(number=1) -> (decimal integer string=w867:string)  [unwired: 1 in]
                            n315 = property on="initial time 2" class="DigNum (strict)"("NumText.Text"=w867) -> ()  [unwired: 2 in, 2 out]
                          }
                        }
                      }
                      frame True {
                        n316 = Increment(x=w886) -> (x+1=w885:i32)
                        n317 = Increment(x=w888) -> (x+1=w887:i32)
                        n318 = stacked-sequence {
                          seq-local: [w935 _] -> [_ w938]
                          tunnel: [w934 _] -> w880
                          frame #0 {
                            n319 = property on="initial time" class="DigNum (strict)"() -> ("NumText.Text"=w937:string)  [unwired: 2 in, 2 out]
                            n320 = Tick Count (ms)() -> (millisecond timer value=w935:u32)
                            n321 = Decimal String To Number(string=w937) -> (number=w936:i32)  [unwired: 2 in, 1 out]
                            n322 = Subtract(x=w935, y=w936) -> (x-y=w934:u32)
                          }
                          frame #1 {
                            n323 = Number To Decimal String(number=w938) -> (decimal integer string=w939:string)  [unwired: 1 in]
                            n324 = property on="initial time" class="DigNum (strict)"("NumText.Text"=w939) -> ()  [unwired: 2 in, 2 out]
                          }
                        }
                        n325 = Current VI's Path() -> (path=w883:path)
                        n326 = Strip Path(path=w883) -> (stripped path=w882:path)  [unwired: 1 out]
                        n327 = Build Path(base path=w882, name or relative path="successful_hit.wav") -> (appended path=w884:path)
                        n328 = call <vilib>:"Play Sound File.vi"("path"=w884) -> ()  [unwired: 9 in, 2 out]
                        n329 = stacked-sequence {
                          tunnel: w879 -> [w891 w902 w913 w923 w932]
                          tunnel: w880 -> [_ w900 _ _ _]
                          tunnel: w878 -> [_ _ w910 _ _]
                          tunnel: [_ _ w911 _ _] -> w877
                          tunnel: w876 -> [_ _ w912 _ _]
                          tunnel: w875 -> [_ w895 _ _ _]
                          tunnel: w872 -> [w892 _ _ _ _]
                          tunnel: [dbl[][] [] _ _ _ _] -> w871
                          frame #0 {
                            n330 = call-poly <vilib>:"Write To Spreadsheet File.vi"("append to file? (new file:F)"=TRUE, "2D data"=w892, "file path (dialog if empty)"=w891) -> ()  [unwired: 5 in, 1 out]
                          }
                          frame #1 {
                            n331 = Greater?(x=w895, y=u32 10000 ("element")) -> (0:w898:bool)
                            n332 = Select(t=1, s=w898, f=w895) -> (s? t:f=w894:i32)
                            n333 = Build Array(w900, w894, u32 0 ("element")) -> (w901:u32[])
                            n334 = call-poly <vilib>:"Write To Spreadsheet File.vi"("append to file? (new file:F)"=TRUE, "1D data"=w901, "file path (dialog if empty)"=w902) -> ()  [unwired: 5 in, 1 out]
                          }
                          frame #2 {
                            w911 = u32 0 ("element")
                            n335 = call "3D_to_Pixels.vi"("Distance_3D"=w910) -> ("Distance_pixels"=w909:dbl)  [unwired: 11 in, 3 out]
                            n336 = Decrement(x=w912) -> (x-1=w905:u32)
                            n337 = Greater?(x=w905, y=u32 10000 ("element")) -> (0:w908:bool)
                            n338 = Select(t=1, s=w908, f=w905) -> (s? t:f=w904:u32)
                            n339 = Build Array(w909, w904, w911) -> (w914:dbl[])
                            n340 = call-poly <vilib>:"Write To Spreadsheet File.vi"("append to file? (new file:F)"=TRUE, "1D data"=w914, "file path (dialog if empty)"=w913) -> ()  [unwired: 5 in, 1 out]
                          }
                          frame #3 {
                            n341 = call "3D_to_Pixels.vi"("X_3D"=0.8 ("element"), "Y_3D"=0.8 ("element"), "Z_3D"=0.8 ("element")) -> ("X_pixels"=w920:dbl, "Y_pixels"=w921:dbl, "Z_pixels"=w922:dbl)  [unwired: 9 in, 1 out]
                            n342 = Build Array(w920, w921, w922) -> (w919:dbl[])
                            n343 = call-poly <vilib>:"Write To Spreadsheet File.vi"("append to file? (new file:F)"=TRUE, "1D data"=w919, "file path (dialog if empty)"=w923) -> ()  [unwired: 5 in, 1 out]
                          }
                          frame #4 {
                            n344 = call "3D_to_Pixels.vi"("X_3D"=-0.8 ("element"), "Y_3D"=-0.8 ("element"), "Z_3D"=-0.8 ("element")) -> ("X_pixels"=w929:dbl, "Y_pixels"=w930:dbl, "Z_pixels"=w931:dbl)  [unwired: 9 in, 1 out]
                            n345 = Build Array(w929, w930, w931) -> (w928:dbl[])
                            n346 = call-poly <vilib>:"Write To Spreadsheet File.vi"("append to file? (new file:F)"=TRUE, "1D data"=w928, "file path (dialog if empty)"=w932) -> ()  [unwired: 5 in, 1 out]
                          }
                        }
                      }
                    }
                  }
                }
              }
              frame 4 {
                n347 = Unbundle(w940) -> ("X_3D"=w955:dbl, "Y_3D"=w954:dbl, "Z_3D"=w953:dbl)
                n348 = call "3D_Session_Data.vi"("Session"=w941) -> ("Radius"=w942:sgl, "min"=w945:dbl, "max"=w944:dbl)  [unwired: 8 in]
                n349 = Less Or Equal?(x=w955, y=w944) -> (x <= y?=w951:bool)
                n350 = Greater Or Equal?(x=w955, y=w945) -> (x >= y?=w952:bool)
                n351 = Less Or Equal?(x=w954, y=w944) -> (x <= y?=w949:bool)
                n352 = Greater Or Equal?(x=w954, y=w945) -> (x >= y?=w950:bool)
                n353 = Less Or Equal?(x=w953, y=w944) -> (x <= y?=w947:bool)
                n354 = Greater Or Equal?(x=w953, y=w945) -> (x >= y?=w948:bool)
                n355 = Build Array(w952, w951, w950, w949, w948, w947) -> (w946:bool[])
                n356 = And Array Elements(Boolean array=w946) -> (logical AND=w943:bool)
                n357 = case shown="True" w943 {
                  tunnel: [T12[] [{"Red"=0.0, "Green"=0.0, "Blue"=0.545, "Alpha"=0.8}, {"Red"=0.0, "Green"=0.0, "Blue"=0.545, "Alpha"=0.8}, {"Red"=0.0, "Green"=1.0, "Blue"=1.0, "Alpha"=0.8}, {"Red"=0.0, "Green"=0.0, "Blue"=0.545, "Alpha"=0.8}, {"Red"=0.0, "Green"=0.0, "Blue"=0.545, "Alpha"=0.8}, {"Red"=0.0, "Green"=0.0, "Blue"=0.545, "Alpha"=0.8}, {"Red"=0.0, "Green"=0.0, "Blue"=0.545, "Alpha"=0.8}, {"Red"=0.0, "Green"=0.0, "Blue"=0.545, "Alpha"=0.8}] ("Array") w1017] -> w972
                  tunnel: [T11 {"Red"=1.0, "Green"=0.0, "Blue"=0.0, "Alpha"=1.0} ("Color") w1016] -> w971
                  tunnel: w970 -> [w976 w1015]
                  tunnel: w969 -> [w985 w1014]
                  tunnel: [w985 w1013] -> w968
                  tunnel: w967 -> [w984 w1012]
                  tunnel: [w984 w1011] -> w966
                  tunnel: w965 -> [_ w1010]
                  tunnel: w942 -> [_ w1009]
                  tunnel: [w983 w1007] -> w964
                  tunnel: w963 -> [w983 w1008]
                  tunnel: w962 -> [w980 w1006]
                  tunnel: w961 -> [w979 w1005]
                  tunnel: [w978 w1006] -> w960
                  tunnel: [w977 w1004] -> w959
                  tunnel: w940 -> [w975 w1003]
                  tunnel: [w975 w1002] -> w958
                  tunnel: w957 -> [w974 w1001]
                  tunnel: [w974 w1000] -> w956
                  frame False {
                    n358 = case shown="False" w976 {
                      tunnel: w980 -> [w988 w999]
                      tunnel: [w987 w998] -> w978
                      tunnel: w979 -> [w990 w997]
                      tunnel: [w989 w997] -> w977
                      frame False {
                        n359 = Greater Than 0?(x=w988) -> (x > 0?=w991:bool)
                        n360 = case shown="True" w991 {
                          tunnel: w990 -> [w993 w996]
                          tunnel: [w993 w995] -> w989
                          tunnel: w988 -> [w992 _]
                          tunnel: [w992 0 ("y")] -> w987
                          frame False {
                          }
                          frame True {
                            n361 = Increment(x=w996) -> (x+1=w995:i32)
                          }
                        }
                      }
                      frame True {
                        n362 = Increment(x=w999) -> (x+1=w998:i32)
                      }
                    }
                    n363 = Number To Decimal String(number=0) -> (decimal integer string=w982:string)  [unwired: 1 in]
                    n364 = property on="initial time 2" class="DigNum (strict)"("NumText.Text"=w982) -> ()  [unwired: 2 in, 2 out]
                  }
                  frame True {
                    n365 = case shown="True" w1015 {
                      tunnel: [T12[] [{"Red"=0.0, "Green"=0.0, "Blue"=0.545, "Alpha"=0.8}, {"Red"=0.0, "Green"=0.0, "Blue"=0.545, "Alpha"=0.8}, {"Red"=0.0, "Green"=0.8, "Blue"=0.0, "Alpha"=0.8}, {"Red"=0.0, "Green"=0.0, "Blue"=0.545, "Alpha"=0.8}, {"Red"=0.0, "Green"=0.0, "Blue"=0.545, "Alpha"=0.8}, {"Red"=0.0, "Green"=0.0, "Blue"=0.545, "Alpha"=0.8}, {"Red"=0.0, "Green"=0.0, "Blue"=0.545, "Alpha"=0.8}, {"Red"=0.0, "Green"=0.0, "Blue"=0.545, "Alpha"=0.8}] ("Array") T12[] [{"Red"=0.0, "Green"=0.0, "Blue"=0.545, "Alpha"=0.8}, {"Red"=0.0, "Green"=0.0, "Blue"=0.545, "Alpha"=0.8}, {"Red"=1.0, "Green"=1.0, "Blue"=0.0, "Alpha"=0.8}, {"Red"=0.0, "Green"=0.0, "Blue"=0.545, "Alpha"=0.8}, {"Red"=0.0, "Green"=0.0, "Blue"=0.545, "Alpha"=0.8}, {"Red"=0.0, "Green"=0.0, "Blue"=0.545, "Alpha"=0.8}, {"Red"=0.0, "Green"=0.0, "Blue"=0.545, "Alpha"=0.8}, {"Red"=0.0, "Green"=0.0, "Blue"=0.545, "Alpha"=0.8}] ("Array")] -> w1017
                      tunnel: [T11 {"Red"=0.0, "Green"=0.8, "Blue"=0.0, "Alpha"=1.0} ("Color") T11 {"Red"=1.0, "Green"=1.0, "Blue"=0.0, "Alpha"=1.0} ("Color")] -> w1016
                      tunnel: w1014 -> [w1028 w1053]
                      tunnel: [w1028 w1052] -> w1013
                      tunnel: w1012 -> [w1027 w1051]
                      tunnel: [w1027 w1050] -> w1011
                      tunnel: w1010 -> [_ w1044]
                      tunnel: w1009 -> [_ w1043]
                      tunnel: w1008 -> [w1023 w1041]
                      tunnel: [w1022 w1042] -> w1007
                      tunnel: w1005 -> [w1021 w1040]
                      tunnel: [w1021 0 ("x")] -> w1004
                      tunnel: w1003 -> [w1020 _]
                      tunnel: [w1020 cluster{dbl, dbl, "y":dbl} {-0.8, 0.8, "y"=0.8}] -> w1002
                      tunnel: w1001 -> [w1019 w1037]
                      tunnel: [w1019 w1036] -> w1000
                      frame False {
                        n366 = property on="initial time 2" class="DigNum (strict)"() -> ("NumText.Text"=w1025:string)  [unwired: 2 in, 2 out]
                        n367 = Decimal String To Number(string=w1025) -> (number=w1024:i32)  [unwired: 2 in, 1 out]
                        n368 = Equal To 0?(x=w1024) -> (x = 0?=w1026:bool)
                        n369 = case shown="False" w1026 {
                          tunnel: w1023 -> [w1030 w1034]
                          tunnel: [w1030 w1033] -> w1022
                          frame False {
                          }
                          frame True {
                            n370 = Increment(x=w1034) -> (x+1=w1033:u32)
                            n371 = Number To Decimal String(number=1) -> (decimal integer string=w1032:string)  [unwired: 1 in]
                            n372 = property on="initial time 2" class="DigNum (strict)"("NumText.Text"=w1032) -> ()  [unwired: 2 in, 2 out]
                          }
                        }
                      }
                      frame True {
                        n373 = Increment(x=w1051) -> (x+1=w1050:i32)
                        n374 = Increment(x=w1053) -> (x+1=w1052:i32)
                        n375 = stacked-sequence {
                          seq-local: [w1100 _] -> [_ w1103]
                          tunnel: [w1099 _] -> w1045
                          frame #0 {
                            n376 = property on="initial time" class="DigNum (strict)"() -> ("NumText.Text"=w1102:string)  [unwired: 2 in, 2 out]
                            n377 = Tick Count (ms)() -> (millisecond timer value=w1100:u32)
                            n378 = Decimal String To Number(string=w1102) -> (number=w1101:i32)  [unwired: 2 in, 1 out]
                            n379 = Subtract(x=w1100, y=w1101) -> (x-y=w1099:u32)
                          }
                          frame #1 {
                            n380 = Number To Decimal String(number=w1103) -> (decimal integer string=w1104:string)  [unwired: 1 in]
                            n381 = property on="initial time" class="DigNum (strict)"("NumText.Text"=w1104) -> ()  [unwired: 2 in, 2 out]
                          }
                        }
                        n382 = Current VI's Path() -> (path=w1048:path)
                        n383 = Strip Path(path=w1048) -> (stripped path=w1047:path)  [unwired: 1 out]
                        n384 = Build Path(base path=w1047, name or relative path="successful_hit.wav") -> (appended path=w1049:path)
                        n385 = call <vilib>:"Play Sound File.vi"("path"=w1049) -> ()  [unwired: 9 in, 2 out]
                        n386 = stacked-sequence {
                          tunnel: w1044 -> [w1056 w1067 w1078 w1088 w1097]
                          tunnel: w1045 -> [_ w1065 _ _ _]
                          tunnel: w1043 -> [_ _ w1074 _ _]
                          tunnel: [_ _ w1076 _ _] -> w1042
                          tunnel: w1041 -> [_ _ w1077 _ _]
                          tunnel: w1040 -> [_ w1060 _ _ _]
                          tunnel: w1037 -> [w1057 _ _ _ _]
                          tunnel: [dbl[][] [] _ _ _ _] -> w1036
                          frame #0 {
                            n387 = call-poly <vilib>:"Write To Spreadsheet File.vi"("append to file? (new file:F)"=TRUE, "2D data"=w1057, "file path (dialog if empty)"=w1056) -> ()  [unwired: 5 in, 1 out]
                          }
                          frame #1 {
                            n388 = Greater?(x=w1060, y=u32 10000 ("element")) -> (0:w1063:bool)
                            n389 = Select(t=1, s=w1063, f=w1060) -> (s? t:f=w1059:i32)
                            n390 = Build Array(w1065, w1059, u32 0 ("element")) -> (w1066:u32[])
                            n391 = call-poly <vilib>:"Write To Spreadsheet File.vi"("append to file? (new file:F)"=TRUE, "1D data"=w1066, "file path (dialog if empty)"=w1067) -> ()  [unwired: 5 in, 1 out]
                          }
                          frame #2 {
                            w1076 = u32 0 ("element")
                            n392 = call "3D_to_Pixels.vi"("Distance_3D"=w1074) -> ("Distance_pixels"=w1075:dbl)  [unwired: 11 in, 3 out]
                            n393 = Decrement(x=w1077) -> (x-1=w1070:u32)
                            n394 = Greater?(x=w1070, y=u32 10000 ("element")) -> (0:w1073:bool)
                            n395 = Select(t=1, s=w1073, f=w1070) -> (s? t:f=w1069:u32)
                            n396 = Build Array(w1075, w1069, w1076) -> (w1080:dbl[])
                            n397 = call-poly <vilib>:"Write To Spreadsheet File.vi"("append to file? (new file:F)"=TRUE, "1D data"=w1080, "file path (dialog if empty)"=w1078) -> ()  [unwired: 5 in, 1 out]
                          }
                          frame #3 {
                            n398 = call "3D_to_Pixels.vi"("X_3D"=-0.8 ("element"), "Y_3D"=-0.8 ("element"), "Z_3D"=-0.8 ("element")) -> ("X_pixels"=w1085:dbl, "Y_pixels"=w1086:dbl, "Z_pixels"=w1087:dbl)  [unwired: 9 in, 1 out]
                            n399 = Build Array(w1085, w1086, w1087) -> (w1084:dbl[])
                            n400 = call-poly <vilib>:"Write To Spreadsheet File.vi"("append to file? (new file:F)"=TRUE, "1D data"=w1084, "file path (dialog if empty)"=w1088) -> ()  [unwired: 5 in, 1 out]
                          }
                          frame #4 {
                            n401 = call "3D_to_Pixels.vi"("X_3D"=0.8 ("element"), "Y_3D"=0.8 ("element"), "Z_3D"=0.8 ("element")) -> ("X_pixels"=w1094:dbl, "Y_pixels"=w1095:dbl, "Z_pixels"=w1096:dbl)  [unwired: 9 in, 1 out]
                            n402 = Build Array(w1094, w1095, w1096) -> (w1093:dbl[])
                            n403 = call-poly <vilib>:"Write To Spreadsheet File.vi"("append to file? (new file:F)"=TRUE, "1D data"=w1093, "file path (dialog if empty)"=w1097) -> ()  [unwired: 5 in, 1 out]
                          }
                        }
                      }
                    }
                  }
                }
              }
              frame 5 {
                n404 = Unbundle(w1107) -> ("X_3D"=w1122:dbl, "Y_3D"=w1121:dbl, "Z_3D"=w1120:dbl)
                n405 = call "3D_Session_Data.vi"("Session"=w1106) -> ("Radius"=w1105:sgl, "min"=w1112:dbl, "max"=w1111:dbl)  [unwired: 8 in]
                n406 = Less Or Equal?(x=w1122, y=w1111) -> (x <= y?=w1118:bool)
                n407 = Greater Or Equal?(x=w1122, y=w1112) -> (x >= y?=w1119:bool)
                n408 = Negate(x=w1111) -> (-x=w1110:dbl)
                n409 = Negate(x=w1112) -> (-x=w1109:dbl)
                n410 = Greater Or Equal?(x=w1121, y=w1110) -> (x >= y?=w1117:bool)
                n411 = Less Or Equal?(x=w1121, y=w1109) -> (x <= y?=w1116:bool)
                n412 = Greater Or Equal?(x=w1120, y=w1110) -> (x >= y?=w1115:bool)
                n413 = Less Or Equal?(x=w1120, y=w1109) -> (x <= y?=w1114:bool)
                n414 = Build Array(w1119, w1118, w1117, w1116, w1115, w1114) -> (w1113:bool[])
                n415 = And Array Elements(Boolean array=w1113) -> (logical AND=w1108:bool)
                n416 = case shown="True" w1108 {
                  tunnel: [T12[] [{"Red"=0.0, "Green"=0.0, "Blue"=0.545, "Alpha"=0.8}, {"Red"=0.0, "Green"=0.0, "Blue"=0.545, "Alpha"=0.8}, {"Red"=0.0, "Green"=0.0, "Blue"=0.545, "Alpha"=0.8}, {"Red"=0.0, "Green"=0.0, "Blue"=0.545, "Alpha"=0.8}, {"Red"=0.0, "Green"=0.0, "Blue"=0.545, "Alpha"=0.8}, {"Red"=0.0, "Green"=1.0, "Blue"=1.0, "Alpha"=0.8}, {"Red"=0.0, "Green"=0.0, "Blue"=0.545, "Alpha"=0.8}, {"Red"=0.0, "Green"=0.0, "Blue"=0.545, "Alpha"=0.8}] ("Array") w1184] -> w1139
                  tunnel: [T11 {"Red"=1.0, "Green"=0.0, "Blue"=0.0, "Alpha"=1.0} ("Color") w1183] -> w1138
                  tunnel: w1137 -> [w1143 w1182]
                  tunnel: w1136 -> [w1152 w1181]
                  tunnel: [w1152 w1180] -> w1135
                  tunnel: w1134 -> [w1151 w1179]
                  tunnel: [w1151 w1178] -> w1133
                  tunnel: w1132 -> [_ w1177]
                  tunnel: w1105 -> [_ w1176]
                  tunnel: [w1150 w1175] -> w1131
                  tunnel: w1130 -> [w1150 w1174]
                  tunnel: w1129 -> [w1147 w1173]
                  tunnel: w1128 -> [w1146 w1172]
                  tunnel: [w1145 w1173] -> w1127
                  tunnel: [w1144 w1171] -> w1126
                  tunnel: w1107 -> [w1142 w1170]
                  tunnel: [w1142 w1169] -> w1125
                  tunnel: w1124 -> [w1141 w1168]
                  tunnel: [w1141 w1167] -> w1123
                  frame False {
                    n417 = case shown="False" w1143 {
                      tunnel: w1147 -> [w1155 w1166]
                      tunnel: [w1154 w1165] -> w1145
                      tunnel: w1146 -> [w1157 w1164]
                      tunnel: [w1156 w1164] -> w1144
                      frame False {
                        n418 = Greater Than 0?(x=w1155) -> (x > 0?=w1158:bool)
                        n419 = case shown="True" w1158 {
                          tunnel: w1157 -> [w1160 w1163]
                          tunnel: [w1160 w1162] -> w1156
                          tunnel: w1155 -> [w1159 _]
                          tunnel: [w1159 0 ("y")] -> w1154
                          frame False {
                          }
                          frame True {
                            n420 = Increment(x=w1163) -> (x+1=w1162:i32)
                          }
                        }
                      }
                      frame True {
                        n421 = Increment(x=w1166) -> (x+1=w1165:i32)
                      }
                    }
                    n422 = Number To Decimal String(number=0) -> (decimal integer string=w1149:string)  [unwired: 1 in]
                    n423 = property on="initial time 2" class="DigNum (strict)"("NumText.Text"=w1149) -> ()  [unwired: 2 in, 2 out]
                  }
                  frame True {
                    n424 = case shown="True" w1182 {
                      tunnel: [T12[] [{"Red"=0.0, "Green"=0.0, "Blue"=0.545, "Alpha"=0.8}, {"Red"=0.0, "Green"=0.0, "Blue"=0.545, "Alpha"=0.8}, {"Red"=0.0, "Green"=0.0, "Blue"=0.545, "Alpha"=0.8}, {"Red"=0.0, "Green"=0.0, "Blue"=0.545, "Alpha"=0.8}, {"Red"=0.0, "Green"=0.0, "Blue"=0.545, "Alpha"=0.8}, {"Red"=0.0, "Green"=0.8, "Blue"=0.0, "Alpha"=0.8}, {"Red"=0.0, "Green"=0.0, "Blue"=0.545, "Alpha"=0.8}, {"Red"=0.0, "Green"=0.0, "Blue"=0.545, "Alpha"=0.8}] ("Array") T12[] [{"Red"=0.0, "Green"=0.0, "Blue"=0.545, "Alpha"=0.8}, {"Red"=0.0, "Green"=0.0, "Blue"=0.545, "Alpha"=0.8}, {"Red"=0.0, "Green"=0.0, "Blue"=0.545, "Alpha"=0.8}, {"Red"=0.0, "Green"=0.0, "Blue"=0.545, "Alpha"=0.8}, {"Red"=0.0, "Green"=0.0, "Blue"=0.545, "Alpha"=0.8}, {"Red"=1.0, "Green"=1.0, "Blue"=0.0, "Alpha"=0.8}, {"Red"=0.0, "Green"=0.0, "Blue"=0.545, "Alpha"=0.8}, {"Red"=0.0, "Green"=0.0, "Blue"=0.545, "Alpha"=0.8}] ("Array")] -> w1184
                      tunnel: [T11 {"Red"=0.0, "Green"=0.8, "Blue"=0.0, "Alpha"=1.0} ("Color") T11 {"Red"=1.0, "Green"=1.0, "Blue"=0.0, "Alpha"=1.0} ("Color")] -> w1183
                      tunnel: w1181 -> [w1195 w1220]
                      tunnel: [w1195 w1219] -> w1180
                      tunnel: w1179 -> [w1194 w1218]
                      tunnel: [w1194 w1217] -> w1178
                      tunnel: w1177 -> [_ w1211]
                      tunnel: w1176 -> [_ w1210]
                      tunnel: [w1189 w1209] -> w1175
                      tunnel: w1174 -> [w1190 w1208]
                      tunnel: w1172 -> [w1188 w1207]
                      tunnel: [w1188 0 ("x")] -> w1171
                      tunnel: w1170 -> [w1187 _]
                      tunnel: [w1187 cluster{dbl, dbl, "y":dbl} {0.8, -0.8, "y"=0.8}] -> w1169
                      tunnel: w1168 -> [w1186 w1204]
                      tunnel: [w1186 w1203] -> w1167
                      frame False {
                        n425 = property on="initial time 2" class="DigNum (strict)"() -> ("NumText.Text"=w1192:string)  [unwired: 2 in, 2 out]
                        n426 = Decimal String To Number(string=w1192) -> (number=w1191:i32)  [unwired: 2 in, 1 out]
                        n427 = Equal To 0?(x=w1191) -> (x = 0?=w1193:bool)
                        n428 = case shown="True" w1193 {
                          tunnel: w1190 -> [w1197 w1201]
                          tunnel: [w1197 w1200] -> w1189
                          frame False {
                          }
                          frame True {
                            n429 = Increment(x=w1201) -> (x+1=w1200:u32)
                            n430 = Number To Decimal String(number=1) -> (decimal integer string=w1199:string)  [unwired: 1 in]
                            n431 = property on="initial time 2" class="DigNum (strict)"("NumText.Text"=w1199) -> ()  [unwired: 2 in, 2 out]
                          }
                        }
                      }
                      frame True {
                        n432 = Increment(x=w1218) -> (x+1=w1217:i32)
                        n433 = Increment(x=w1220) -> (x+1=w1219:i32)
                        n434 = stacked-sequence {
                          seq-local: [w1267 _] -> [_ w1270]
                          tunnel: [w1266 _] -> w1212
                          frame #0 {
                            n435 = property on="initial time" class="DigNum (strict)"() -> ("NumText.Text"=w1269:string)  [unwired: 2 in, 2 out]
                            n436 = Tick Count (ms)() -> (millisecond timer value=w1267:u32)
                            n437 = Decimal String To Number(string=w1269) -> (number=w1268:i32)  [unwired: 2 in, 1 out]
                            n438 = Subtract(x=w1267, y=w1268) -> (x-y=w1266:u32)
                          }
                          frame #1 {
                            n439 = Number To Decimal String(number=w1270) -> (decimal integer string=w1271:string)  [unwired: 1 in]
                            n440 = property on="initial time" class="DigNum (strict)"("NumText.Text"=w1271) -> ()  [unwired: 2 in, 2 out]
                          }
                        }
                        n441 = Current VI's Path() -> (path=w1215:path)
                        n442 = Strip Path(path=w1215) -> (stripped path=w1214:path)  [unwired: 1 out]
                        n443 = Build Path(base path=w1214, name or relative path="successful_hit.wav") -> (appended path=w1216:path)
                        n444 = call <vilib>:"Play Sound File.vi"("path"=w1216) -> ()  [unwired: 9 in, 2 out]
                        n445 = stacked-sequence {
                          tunnel: w1211 -> [w1223 w1234 w1245 w1255 w1264]
                          tunnel: w1212 -> [_ w1232 _ _ _]
                          tunnel: w1210 -> [_ _ w1242 _ _]
                          tunnel: [_ _ w1243 _ _] -> w1209
                          tunnel: w1208 -> [_ _ w1244 _ _]
                          tunnel: w1207 -> [_ w1227 _ _ _]
                          tunnel: w1204 -> [w1224 _ _ _ _]
                          tunnel: [dbl[][] [] _ _ _ _] -> w1203
                          frame #0 {
                            n446 = call-poly <vilib>:"Write To Spreadsheet File.vi"("append to file? (new file:F)"=TRUE, "2D data"=w1224, "file path (dialog if empty)"=w1223) -> ()  [unwired: 5 in, 1 out]
                          }
                          frame #1 {
                            n447 = Greater?(x=w1227, y=u32 10000 ("element")) -> (0:w1230:bool)
                            n448 = Select(t=1, s=w1230, f=w1227) -> (s? t:f=w1226:i32)
                            n449 = Build Array(w1232, w1226, u32 0 ("element")) -> (w1233:u32[])
                            n450 = call-poly <vilib>:"Write To Spreadsheet File.vi"("append to file? (new file:F)"=TRUE, "1D data"=w1233, "file path (dialog if empty)"=w1234) -> ()  [unwired: 5 in, 1 out]
                          }
                          frame #2 {
                            w1243 = u32 0 ("element")
                            n451 = call "3D_to_Pixels.vi"("Distance_3D"=w1242) -> ("Distance_pixels"=w1241:dbl)  [unwired: 11 in, 3 out]
                            n452 = Decrement(x=w1244) -> (x-1=w1237:u32)
                            n453 = Greater?(x=w1237, y=u32 10000 ("element")) -> (0:w1240:bool)
                            n454 = Select(t=1, s=w1240, f=w1237) -> (s? t:f=w1236:u32)
                            n455 = Build Array(w1241, w1236, w1243) -> (w1246:dbl[])
                            n456 = call-poly <vilib>:"Write To Spreadsheet File.vi"("append to file? (new file:F)"=TRUE, "1D data"=w1246, "file path (dialog if empty)"=w1245) -> ()  [unwired: 5 in, 1 out]
                          }
                          frame #3 {
                            n457 = call "3D_to_Pixels.vi"("X_3D"=-0.8 ("element"), "Y_3D"=0.8 ("element"), "Z_3D"=0.8 ("element")) -> ("X_pixels"=w1252:dbl, "Y_pixels"=w1253:dbl, "Z_pixels"=w1254:dbl)  [unwired: 9 in, 1 out]
                            n458 = Build Array(w1252, w1253, w1254) -> (w1251:dbl[])
                            n459 = call-poly <vilib>:"Write To Spreadsheet File.vi"("append to file? (new file:F)"=TRUE, "1D data"=w1251, "file path (dialog if empty)"=w1255) -> ()  [unwired: 5 in, 1 out]
                          }
                          frame #4 {
                            n460 = call "3D_to_Pixels.vi"("X_3D"=0.8 ("element"), "Y_3D"=-0.8 ("element"), "Z_3D"=-0.8 ("element")) -> ("X_pixels"=w1261:dbl, "Y_pixels"=w1262:dbl, "Z_pixels"=w1263:dbl)  [unwired: 9 in, 1 out]
                            n461 = Build Array(w1261, w1262, w1263) -> (w1260:dbl[])
                            n462 = call-poly <vilib>:"Write To Spreadsheet File.vi"("append to file? (new file:F)"=TRUE, "1D data"=w1260, "file path (dialog if empty)"=w1264) -> ()  [unwired: 5 in, 1 out]
                          }
                        }
                      }
                    }
                  }
                }
              }
              frame 6 {
                n463 = Unbundle(w1273) -> ("X_3D"=w1289:dbl, "Y_3D"=w1288:dbl, "Z_3D"=w1287:dbl)
                n464 = call "3D_Session_Data.vi"("Session"=w1274) -> ("Radius"=w1272:sgl, "min"=w1279:dbl, "max"=w1278:dbl)  [unwired: 8 in]
                n465 = Less Or Equal?(x=w1288, y=w1278) -> (x <= y?=w1283:bool)
                n466 = Greater Or Equal?(x=w1288, y=w1279) -> (x >= y?=w1284:bool)
                n467 = Negate(x=w1278) -> (-x=w1277:dbl)
                n468 = Negate(x=w1279) -> (-x=w1276:dbl)
                n469 = Greater Or Equal?(x=w1289, y=w1277) -> (x >= y?=w1286:bool)
                n470 = Less Or Equal?(x=w1289, y=w1276) -> (x <= y?=w1285:bool)
                n471 = Greater Or Equal?(x=w1287, y=w1277) -> (x >= y?=w1282:bool)
                n472 = Less Or Equal?(x=w1287, y=w1276) -> (x <= y?=w1281:bool)
                n473 = Build Array(w1286, w1285, w1284, w1283, w1282, w1281) -> (w1280:bool[])
                n474 = And Array Elements(Boolean array=w1280) -> (logical AND=w1275:bool)
                n475 = case shown="True" w1275 {
                  tunnel: [T12[] [{"Red"=0.0, "Green"=0.0, "Blue"=0.545, "Alpha"=0.8}, {"Red"=0.0, "Green"=0.0, "Blue"=0.545, "Alpha"=0.8}, {"Red"=0.0, "Green"=0.0, "Blue"=0.545, "Alpha"=0.8}, {"Red"=0.0, "Green"=0.0, "Blue"=0.545, "Alpha"=0.8}, {"Red"=0.0, "Green"=0.0, "Blue"=0.545, "Alpha"=0.8}, {"Red"=0.0, "Green"=0.0, "Blue"=0.545, "Alpha"=0.8}, {"Red"=0.0, "Green"=1.0, "Blue"=1.0, "Alpha"=0.8}, {"Red"=0.0, "Green"=0.0, "Blue"=0.545, "Alpha"=0.8}] ("Array") w1351] -> w1306
                  tunnel: [T11 {"Red"=1.0, "Green"=0.0, "Blue"=0.0, "Alpha"=1.0} ("Color") w1350] -> w1305
                  tunnel: w1304 -> [w1314 w1349]
                  tunnel: w1303 -> [w1319 w1348]
                  tunnel: [w1319 w1347] -> w1302
                  tunnel: w1301 -> [w1318 w1346]
                  tunnel: [w1318 w1345] -> w1300
                  tunnel: w1299 -> [_ w1344]
                  tunnel: w1272 -> [_ w1343]
                  tunnel: [w1317 w1342] -> w1298
                  tunnel: w1297 -> [w1317 w1341]
                  tunnel: w1296 -> [w1313 w1340]
                  tunnel: w1295 -> [w1312 w1339]
                  tunnel: [w1311 w1340] -> w1294
                  tunnel: [w1310 w1338] -> w1293
                  tunnel: w1273 -> [w1309 w1337]
                  tunnel: [w1309 w1336] -> w1292
                  tunnel: w1291 -> [w1308 w1335]
                  tunnel: [w1308 w1334] -> w1290
                  frame False {
                    n476 = case shown="False" w1314 {
                      tunnel: w1313 -> [w1322 w1333]
                      tunnel: [w1321 w1332] -> w1311
                      tunnel: w1312 -> [w1324 w1331]
                      tunnel: [w1323 w1331] -> w1310
                      frame False {
                        n477 = Greater Than 0?(x=w1322) -> (x > 0?=w1325:bool)
                        n478 = case shown="False" w1325 {
                          tunnel: w1324 -> [w1327 w1330]
                          tunnel: [w1327 w1329] -> w1323
                          tunnel: w1322 -> [w1326 _]
                          tunnel: [w1326 0 ("y")] -> w1321
                          frame False {
                          }
                          frame True {
                            n479 = Increment(x=w1330) -> (x+1=w1329:i32)
                          }
                        }
                      }
                      frame True {
                        n480 = Increment(x=w1333) -> (x+1=w1332:i32)
                      }
                    }
                    n481 = Number To Decimal String(number=0) -> (decimal integer string=w1316:string)  [unwired: 1 in]
                    n482 = property on="initial time 2" class="DigNum (strict)"("NumText.Text"=w1316) -> ()  [unwired: 2 in, 2 out]
                  }
                  frame True {
                    n483 = case shown="True" w1349 {
                      tunnel: [T12[] [{"Red"=0.0, "Green"=0.0, "Blue"=0.545, "Alpha"=0.8}, {"Red"=0.0, "Green"=0.0, "Blue"=0.545, "Alpha"=0.8}, {"Red"=0.0, "Green"=0.0, "Blue"=0.545, "Alpha"=0.8}, {"Red"=0.0, "Green"=0.0, "Blue"=0.545, "Alpha"=0.8}, {"Red"=0.0, "Green"=0.0, "Blue"=0.545, "Alpha"=0.8}, {"Red"=0.0, "Green"=0.0, "Blue"=0.545, "Alpha"=0.8}, {"Red"=0.0, "Green"=0.8, "Blue"=0.0, "Alpha"=0.8}, {"Red"=0.0, "Green"=0.0, "Blue"=0.545, "Alpha"=0.8}] ("Array") T12[] [{"Red"=0.0, "Green"=0.0, "Blue"=0.545, "Alpha"=0.8}, {"Red"=0.0, "Green"=0.0, "Blue"=0.545, "Alpha"=0.8}, {"Red"=0.0, "Green"=0.0, "Blue"=0.545, "Alpha"=0.8}, {"Red"=0.0, "Green"=0.0, "Blue"=0.545, "Alpha"=0.8}, {"Red"=0.0, "Green"=0.0, "Blue"=0.545, "Alpha"=0.8}, {"Red"=0.0, "Green"=0.0, "Blue"=0.545, "Alpha"=0.8}, {"Red"=1.0, "Green"=1.0, "Blue"=0.0, "Alpha"=0.8}, {"Red"=0.0, "Green"=0.0, "Blue"=0.545, "Alpha"=0.8}] ("Array")] -> w1351
                      tunnel: [T11 {"Red"=0.0, "Green"=0.8, "Blue"=0.0, "Alpha"=1.0} ("Color") T11 {"Red"=1.0, "Green"=1.0, "Blue"=0.0, "Alpha"=1.0} ("Color")] -> w1350
                      tunnel: w1348 -> [w1362 w1387]
                      tunnel: [w1362 w1386] -> w1347
                      tunnel: w1346 -> [w1361 w1385]
                      tunnel: [w1361 w1384] -> w1345
                      tunnel: w1344 -> [_ w1378]
                      tunnel: w1343 -> [_ w1377]
                      tunnel: [w1357 w1376] -> w1342
                      tunnel: w1341 -> [w1356 w1375]
                      tunnel: w1339 -> [w1355 w1374]
                      tunnel: [w1355 0 ("x")] -> w1338
                      tunnel: w1337 -> [w1354 _]
                      tunnel: [w1354 cluster{dbl, dbl, "y":dbl} {0.8, 0.8, "y"=-0.8}] -> w1336
                      tunnel: w1335 -> [w1353 w1371]
                      tunnel: [w1353 w1370] -> w1334
                      frame False {
                        n484 = property on="initial time 2" class="DigNum (strict)"() -> ("NumText.Text"=w1359:string)  [unwired: 2 in, 2 out]
                        n485 = Decimal String To Number(string=w1359) -> (number=w1358:i32)  [unwired: 2 in, 1 out]
                        n486 = Equal To 0?(x=w1358) -> (x = 0?=w1360:bool)
                        n487 = case shown="True" w1360 {
                          tunnel: w1356 -> [w1364 w1368]
                          tunnel: [w1364 w1367] -> w1357
                          frame False {
                          }
                          frame True {
                            n488 = Increment(x=w1368) -> (x+1=w1367:u32)
                            n489 = Number To Decimal String(number=1) -> (decimal integer string=w1366:string)  [unwired: 1 in]
                            n490 = property on="initial time 2" class="DigNum (strict)"("NumText.Text"=w1366) -> ()  [unwired: 2 in, 2 out]
                          }
                        }
                      }
                      frame True {
                        n491 = Increment(x=w1385) -> (x+1=w1384:i32)
                        n492 = Increment(x=w1387) -> (x+1=w1386:i32)
                        n493 = stacked-sequence {
                          seq-local: [w1434 _] -> [_ w1437]
                          tunnel: [w1433 _] -> w1379
                          frame #0 {
                            n494 = property on="initial time" class="DigNum (strict)"() -> ("NumText.Text"=w1436:string)  [unwired: 2 in, 2 out]
                            n495 = Tick Count (ms)() -> (millisecond timer value=w1434:u32)
                            n496 = Decimal String To Number(string=w1436) -> (number=w1435:i32)  [unwired: 2 in, 1 out]
                            n497 = Subtract(x=w1434, y=w1435) -> (x-y=w1433:u32)
                          }
                          frame #1 {
                            n498 = Number To Decimal String(number=w1437) -> (decimal integer string=w1438:string)  [unwired: 1 in]
                            n499 = property on="initial time" class="DigNum (strict)"("NumText.Text"=w1438) -> ()  [unwired: 2 in, 2 out]
                          }
                        }
                        n500 = Current VI's Path() -> (path=w1382:path)
                        n501 = Strip Path(path=w1382) -> (stripped path=w1381:path)  [unwired: 1 out]
                        n502 = Build Path(base path=w1381, name or relative path="successful_hit.wav") -> (appended path=w1383:path)
                        n503 = call <vilib>:"Play Sound File.vi"("path"=w1383) -> ()  [unwired: 9 in, 2 out]
                        n504 = stacked-sequence {
                          tunnel: w1378 -> [w1390 w1401 w1412 w1422 w1431]
                          tunnel: w1379 -> [_ w1399 _ _ _]
                          tunnel: w1377 -> [_ _ w1408 _ _]
                          tunnel: [_ _ w1410 _ _] -> w1376
                          tunnel: w1375 -> [_ _ w1411 _ _]
                          tunnel: w1374 -> [_ w1394 _ _ _]
                          tunnel: w1371 -> [w1391 _ _ _ _]
                          tunnel: [dbl[][] [] _ _ _ _] -> w1370
                          frame #0 {
                            n505 = call-poly <vilib>:"Write To Spreadsheet File.vi"("append to file? (new file:F)"=TRUE, "2D data"=w1391, "file path (dialog if empty)"=w1390) -> ()  [unwired: 5 in, 1 out]
                          }
                          frame #1 {
                            n506 = Greater?(x=w1394, y=u32 10000 ("element")) -> (0:w1397:bool)
                            n507 = Select(t=1, s=w1397, f=w1394) -> (s? t:f=w1393:i32)
                            n508 = Build Array(w1399, w1393, u32 0 ("element")) -> (w1400:u32[])
                            n509 = call-poly <vilib>:"Write To Spreadsheet File.vi"("append to file? (new file:F)"=TRUE, "1D data"=w1400, "file path (dialog if empty)"=w1401) -> ()  [unwired: 5 in, 1 out]
                          }
                          frame #2 {
                            w1410 = u32 0 ("element")
                            n510 = call "3D_to_Pixels.vi"("Distance_3D"=w1408) -> ("Distance_pixels"=w1409:dbl)  [unwired: 11 in, 3 out]
                            n511 = Decrement(x=w1411) -> (x-1=w1404:u32)
                            n512 = Greater?(x=w1404, y=u32 10000 ("element")) -> (0:w1407:bool)
                            n513 = Select(t=1, s=w1407, f=w1404) -> (s? t:f=w1403:u32)
                            n514 = Build Array(w1409, w1403, w1410) -> (w1413:dbl[])
                            n515 = call-poly <vilib>:"Write To Spreadsheet File.vi"("append to file? (new file:F)"=TRUE, "1D data"=w1413, "file path (dialog if empty)"=w1412) -> ()  [unwired: 5 in, 1 out]
                          }
                          frame #3 {
                            n516 = call "3D_to_Pixels.vi"("X_3D"=0.8 ("element"), "Y_3D"=-0.8 ("element"), "Z_3D"=0.8 ("element")) -> ("X_pixels"=w1419:dbl, "Y_pixels"=w1420:dbl, "Z_pixels"=w1421:dbl)  [unwired: 9 in, 1 out]
                            n517 = Build Array(w1419, w1420, w1421) -> (w1418:dbl[])
                            n518 = call-poly <vilib>:"Write To Spreadsheet File.vi"("append to file? (new file:F)"=TRUE, "1D data"=w1418, "file path (dialog if empty)"=w1422) -> ()  [unwired: 5 in, 1 out]
                          }
                          frame #4 {
                            n519 = call "3D_to_Pixels.vi"("X_3D"=-0.8 ("element"), "Y_3D"=0.8 ("element"), "Z_3D"=-0.8 ("element")) -> ("X_pixels"=w1428:dbl, "Y_pixels"=w1429:dbl, "Z_pixels"=w1430:dbl)  [unwired: 9 in, 1 out]
                            n520 = Build Array(w1428, w1429, w1430) -> (w1427:dbl[])
                            n521 = call-poly <vilib>:"Write To Spreadsheet File.vi"("append to file? (new file:F)"=TRUE, "1D data"=w1427, "file path (dialog if empty)"=w1431) -> ()  [unwired: 5 in, 1 out]
                          }
                        }
                      }
                    }
                  }
                }
              }
              frame 7, Default {
                n522 = Unbundle(w1441) -> ("X_3D"=w1456:dbl, "Y_3D"=w1455:dbl, "Z_3D"=w1454:dbl)
                n523 = call "3D_Session_Data.vi"("Session"=w1440) -> ("Radius"=w1439:sgl, "min"=w1444:dbl, "max"=w1443:dbl)  [unwired: 8 in]
                n524 = Less Or Equal?(x=w1454, y=w1443) -> (x <= y?=w1448:bool)
                n525 = Greater Or Equal?(x=w1454, y=w1444) -> (x >= y?=w1449:bool)
                n526 = Negate(x=w1443) -> (-x=w1446:dbl)
                n527 = Negate(x=w1444) -> (-x=w1445:dbl)
                n528 = Greater Or Equal?(x=w1456, y=w1446) -> (x >= y?=w1453:bool)
                n529 = Less Or Equal?(x=w1456, y=w1445) -> (x <= y?=w1452:bool)
                n530 = Greater Or Equal?(x=w1455, y=w1446) -> (x >= y?=w1451:bool)
                n531 = Less Or Equal?(x=w1455, y=w1445) -> (x <= y?=w1450:bool)
                n532 = Build Array(w1453, w1452, w1451, w1450, w1449, w1448) -> (w1447:bool[])
                n533 = And Array Elements(Boolean array=w1447) -> (logical AND=w1442:bool)
                n534 = case shown="True" w1442 {
                  tunnel: [T12[] [{"Red"=0.0, "Green"=0.0, "Blue"=0.545, "Alpha"=0.8}, {"Red"=0.0, "Green"=1.0, "Blue"=1.0, "Alpha"=0.8}, {"Red"=0.0, "Green"=0.0, "Blue"=0.545, "Alpha"=0.8}, {"Red"=0.0, "Green"=0.0, "Blue"=0.545, "Alpha"=0.8}, {"Red"=0.0, "Green"=0.0, "Blue"=0.545, "Alpha"=0.8}, {"Red"=0.0, "Green"=0.0, "Blue"=0.545, "Alpha"=0.8}, {"Red"=0.0, "Green"=0.0, "Blue"=0.545, "Alpha"=0.8}, {"Red"=0.0, "Green"=0.0, "Blue"=0.545, "Alpha"=0.8}] ("Array") w1518] -> w1473
                  tunnel: [T11 {"Red"=1.0, "Green"=0.0, "Blue"=0.0, "Alpha"=1.0} ("Color") w1517] -> w1472
                  tunnel: w1471 -> [w1477 w1516]
                  tunnel: w1470 -> [w1486 w1515]
                  tunnel: [w1486 w1514] -> w1469
                  tunnel: w1468 -> [w1485 w1513]
                  tunnel: [w1485 w1512] -> w1467
                  tunnel: w1466 -> [_ w1511]
                  tunnel: w1439 -> [_ w1510]
                  tunnel: w1465 -> [w1484 w1509]
                  tunnel: [w1484 w1508] -> w1464
                  tunnel: w1463 -> [w1481 w1507]
                  tunnel: w1462 -> [w1480 w1506]
                  tunnel: [w1479 w1507] -> w1461
                  tunnel: [w1478 w1505] -> w1460
                  tunnel: w1441 -> [w1476 w1504]
                  tunnel: [w1476 w1503] -> w1459
                  tunnel: w1458 -> [w1475 w1502]
                  tunnel: [w1475 w1501] -> w1457
                  frame False {
                    n535 = case shown="False" w1477 {
                      tunnel: w1481 -> [w1489 w1500]
                      tunnel: [w1488 w1499] -> w1479
                      tunnel: w1480 -> [w1491 w1498]
                      tunnel: [w1490 w1498] -> w1478
                      frame False {
                        n536 = Greater Than 0?(x=w1489) -> (x > 0?=w1492:bool)
                        n537 = case shown="True" w1492 {
                          tunnel: w1491 -> [w1494 w1497]
                          tunnel: [w1494 w1496] -> w1490
                          tunnel: w1489 -> [w1493 _]
                          tunnel: [w1493 0 ("y")] -> w1488
                          frame False {
                          }
                          frame True {
                            n538 = Increment(x=w1497) -> (x+1=w1496:i32)
                          }
                        }
                      }
                      frame True {
                        n539 = Increment(x=w1500) -> (x+1=w1499:i32)
                      }
                    }
                    n540 = Number To Decimal String(number=0) -> (decimal integer string=w1483:string)  [unwired: 1 in]
                    n541 = property on="initial time 2" class="DigNum (strict)"("NumText.Text"=w1483) -> ()  [unwired: 2 in, 2 out]
                  }
                  frame True {
                    n542 = case shown="True" w1516 {
                      tunnel: [T12[] [{"Red"=0.0, "Green"=0.0, "Blue"=0.545, "Alpha"=0.8}, {"Red"=0.0, "Green"=0.8, "Blue"=0.0, "Alpha"=0.8}, {"Red"=0.0, "Green"=0.0, "Blue"=0.545, "Alpha"=0.8}, {"Red"=0.0, "Green"=0.0, "Blue"=0.545, "Alpha"=0.8}, {"Red"=0.0, "Green"=0.0, "Blue"=0.545, "Alpha"=0.8}, {"Red"=0.0, "Green"=0.0, "Blue"=0.545, "Alpha"=0.8}, {"Red"=0.0, "Green"=0.0, "Blue"=0.545, "Alpha"=0.8}, {"Red"=0.0, "Green"=0.0, "Blue"=0.545, "Alpha"=0.8}] ("Array") T12[] [{"Red"=0.0, "Green"=0.0, "Blue"=0.545, "Alpha"=0.8}, {"Red"=1.0, "Green"=1.0, "Blue"=0.0, "Alpha"=0.8}, {"Red"=0.0, "Green"=0.0, "Blue"=0.545, "Alpha"=0.8}, {"Red"=0.0, "Green"=0.0, "Blue"=0.545, "Alpha"=0.8}, {"Red"=0.0, "Green"=0.0, "Blue"=0.545, "Alpha"=0.8}, {"Red"=0.0, "Green"=0.0, "Blue"=0.545, "Alpha"=0.8}, {"Red"=0.0, "Green"=0.0, "Blue"=0.545, "Alpha"=0.8}, {"Red"=0.0, "Green"=0.0, "Blue"=0.545, "Alpha"=0.8}] ("Array")] -> w1518
                      tunnel: [T11 {"Red"=0.0, "Green"=0.8, "Blue"=0.0, "Alpha"=1.0} ("Color") T11 {"Red"=1.0, "Green"=1.0, "Blue"=0.0, "Alpha"=1.0} ("Color")] -> w1517
                      tunnel: w1515 -> [w1529 w1554]
                      tunnel: [w1529 w1553] -> w1514
                      tunnel: w1513 -> [w1528 w1552]
                      tunnel: [w1528 w1551] -> w1512
                      tunnel: w1511 -> [_ w1545]
                      tunnel: w1510 -> [_ w1544]
                      tunnel: w1509 -> [w1523 w1543]
                      tunnel: [w1524 w1542] -> w1508
                      tunnel: w1506 -> [w1522 w1541]
                      tunnel: [w1522 0 ("x")] -> w1505
                      tunnel: w1504 -> [w1521 _]
                      tunnel: [w1521 cluster{dbl, dbl, "y":dbl} {-0.8, -0.8, "y"=0.8}] -> w1503
                      tunnel: w1502 -> [w1520 w1538]
                      tunnel: [w1520 w1537] -> w1501
                      frame False {
                        n543 = property on="initial time 2" class="DigNum (strict)"() -> ("NumText.Text"=w1526:string)  [unwired: 2 in, 2 out]
                        n544 = Decimal String To Number(string=w1526) -> (number=w1525:i32)  [unwired: 2 in, 1 out]
                        n545 = Equal To 0?(x=w1525) -> (x = 0?=w1527:bool)
                        n546 = case shown="True" w1527 {
                          tunnel: w1523 -> [w1531 w1535]
                          tunnel: [w1531 w1534] -> w1524
                          frame False {
                          }
                          frame True {
                            n547 = Increment(x=w1535) -> (x+1=w1534:u32)
                            n548 = Number To Decimal String(number=1) -> (decimal integer string=w1533:string)  [unwired: 1 in]
                            n549 = property on="initial time 2" class="DigNum (strict)"("NumText.Text"=w1533) -> ()  [unwired: 2 in, 2 out]
                          }
                        }
                      }
                      frame True {
                        n550 = Increment(x=w1552) -> (x+1=w1551:i32)
                        n551 = Increment(x=w1554) -> (x+1=w1553:i32)
                        n552 = stacked-sequence {
                          seq-local: [w1601 _] -> [_ w1604]
                          tunnel: [w1600 _] -> w1546
                          frame #0 {
                            n553 = property on="initial time" class="DigNum (strict)"() -> ("NumText.Text"=w1603:string)  [unwired: 2 in, 2 out]
                            n554 = Tick Count (ms)() -> (millisecond timer value=w1601:u32)
                            n555 = Decimal String To Number(string=w1603) -> (number=w1602:i32)  [unwired: 2 in, 1 out]
                            n556 = Subtract(x=w1601, y=w1602) -> (x-y=w1600:u32)
                          }
                          frame #1 {
                            n557 = Number To Decimal String(number=w1604) -> (decimal integer string=w1605:string)  [unwired: 1 in]
                            n558 = property on="initial time" class="DigNum (strict)"("NumText.Text"=w1605) -> ()  [unwired: 2 in, 2 out]
                          }
                        }
                        n559 = Current VI's Path() -> (path=w1549:path)
                        n560 = Strip Path(path=w1549) -> (stripped path=w1548:path)  [unwired: 1 out]
                        n561 = Build Path(base path=w1548, name or relative path="successful_hit.wav") -> (appended path=w1550:path)
                        n562 = call <vilib>:"Play Sound File.vi"("path"=w1550) -> ()  [unwired: 9 in, 2 out]
                        n563 = stacked-sequence {
                          tunnel: w1545 -> [w1557 w1568 w1579 w1589 w1598]
                          tunnel: w1546 -> [_ w1566 _ _ _]
                          tunnel: w1544 -> [_ _ w1575 _ _]
                          tunnel: w1543 -> [_ _ w1578 _ _]
                          tunnel: [_ _ w1577 _ _] -> w1542
                          tunnel: w1541 -> [_ w1561 _ _ _]
                          tunnel: w1538 -> [w1558 _ _ _ _]
                          tunnel: [dbl[][] [] _ _ _ _] -> w1537
                          frame #0 {
                            n564 = call-poly <vilib>:"Write To Spreadsheet File.vi"("append to file? (new file:F)"=TRUE, "2D data"=w1558, "file path (dialog if empty)"=w1557) -> ()  [unwired: 5 in, 1 out]
                          }
                          frame #1 {
                            n565 = Greater?(x=w1561, y=u32 10000 ("element")) -> (0:w1564:bool)
                            n566 = Select(t=1, s=w1564, f=w1561) -> (s? t:f=w1560:i32)
                            n567 = Build Array(w1566, w1560, u32 0 ("element")) -> (w1567:u32[])
                            n568 = call-poly <vilib>:"Write To Spreadsheet File.vi"("append to file? (new file:F)"=TRUE, "1D data"=w1567, "file path (dialog if empty)"=w1568) -> ()  [unwired: 5 in, 1 out]
                          }
                          frame #2 {
                            w1577 = u32 0 ("element")
                            n569 = call "3D_to_Pixels.vi"("Distance_3D"=w1575) -> ("Distance_pixels"=w1576:dbl)  [unwired: 11 in, 3 out]
                            n570 = Decrement(x=w1578) -> (x-1=w1571:u32)
                            n571 = Greater?(x=w1571, y=u32 10000 ("element")) -> (0:w1574:bool)
                            n572 = Select(t=1, s=w1574, f=w1571) -> (s? t:f=w1570:u32)
                            n573 = Build Array(w1576, w1570, w1577) -> (w1580:dbl[])
                            n574 = call-poly <vilib>:"Write To Spreadsheet File.vi"("append to file? (new file:F)"=TRUE, "1D data"=w1580, "file path (dialog if empty)"=w1579) -> ()  [unwired: 5 in, 1 out]
                          }
                          frame #3 {
                            n575 = call "3D_to_Pixels.vi"("X_3D"=0.8 ("element"), "Y_3D"=0.8 ("element"), "Z_3D"=-0.8 ("element")) -> ("X_pixels"=w1586:dbl, "Y_pixels"=w1587:dbl, "Z_pixels"=w1588:dbl)  [unwired: 9 in, 1 out]
                            n576 = Build Array(w1586, w1587, w1588) -> (w1585:dbl[])
                            n577 = call-poly <vilib>:"Write To Spreadsheet File.vi"("append to file? (new file:F)"=TRUE, "1D data"=w1585, "file path (dialog if empty)"=w1589) -> ()  [unwired: 5 in, 1 out]
                          }
                          frame #4 {
                            n578 = call "3D_to_Pixels.vi"("X_3D"=-0.8 ("element"), "Y_3D"=-0.8 ("element"), "Z_3D"=0.8 ("element")) -> ("X_pixels"=w1595:dbl, "Y_pixels"=w1596:dbl, "Z_pixels"=w1597:dbl)  [unwired: 9 in, 1 out]
                            n579 = Build Array(w1595, w1596, w1597) -> (w1594:dbl[])
                            n580 = call-poly <vilib>:"Write To Spreadsheet File.vi"("append to file? (new file:F)"=TRUE, "1D data"=w1594, "file path (dialog if empty)"=w1598) -> ()  [unwired: 5 in, 1 out]
                          }
                        }
                      }
                    }
                  }
                }
              }
            }
          }
        }
        n581 = for {
          tunnel: w193 -> [w210] mode=indexing
          tunnel: w192 -> [w213] mode=indexing
          tunnel: w190 -> [w212]
          tunnel: w189 -> [w211] mode=indexing
          n582 = property class="SceneSphere"(reference=w211, "Radius"=w212) -> ()  [unwired: 1 in, 2 out]
          n583 = property class="SceneObject"(reference=w210, "Material.Diffuse"=w213) -> ()  [unwired: 1 in, 2 out]
        }
        n584 = property class="SceneSphere"(reference=w191, "Radius"=w190) -> ()  [unwired: 1 in, 2 out]
        n585 = call <vilib>:"Set Translation.vi"("Translation"=w148, "Scene Object"=w196) -> ("Translated Object"=w194:refnum<vi>)  [unwired: 8 in, 1 out]
        n586 = property class="SceneObject"(reference=w194, "Material.Diffuse"=w195) -> ()  [unwired: 1 in, 2 out]
        n587 = Bundle("average Y"=w125, "average X"=w126, "average Z"=w124) -> (w154:T20)  [unwired: 1 in]
        n588 = node-c288() -> ()  [unwired: 1 in, 1 out]
        "3D Picture" <- w197
      }
      n589 = node-c288(w119) -> ()  [unwired: 1 out]
      n590 = call "Dispose Kinect.vi"("error in (no error)"=w51, "Queues In"=w49, "References"=w50) -> ("error out"=w52:errorcluster)  [unwired: 2 in]
      n591 = call-poly <vilib>:"Close Input Device.vi"("error in (no error)"=w61, "device ID"=w59) -> ()  [unwired: 8 in, 1 out]
      n592 = call "IMAQ Dispose"("All Images? (No)"=TRUE, "error in (no error)"=w52) -> ("error out"=w53:errorcluster)  [unwired: 4 in]
      n593 = call <vilib>:"Simple Error Handler.vi"("error in (no error)"=w53) -> ()  [unwired: 4 in, 5 out]
    }
    frame #2 {
      n594 = call "Time Delay2"() -> ()  [unwired: 11 in, 1 out]
    }
  }
  n595 = node-c288() -> (w2:T8)  [unwired: 4 in]
  n596 = timed-loop {
    shift-right: [w1615] -> _
    shift-left: _ -> [w1614]
    timing: w2 -> [_]
    timing-out: [_] -> w1
    stop <- w1613 stop-if-true
    n597 = node-c288() -> ()  [unwired: 1 in, 1 out]
    n598 = call "Acquire Sound"() -> ("Data"=w1621:dynamicdata)  [unwired: 18 in, 1 out]
    n599 = call "Tone Measurements"("Signals"=w1621) -> ("Amplitude"=w1620:dynamicdata)  [unwired: 9 in, 1 out]
    n600 = Greater?(x=w1620, y=0.105) -> (0:w1618:dynamicdata)
    n601 = call "Convert from Dynamic Data"("Dynamic Data Type"=w1618) -> ("Scalar"=w1615:bool)  [unwired: 3 in]
    n602 = Not(x=w1614) -> (.not. x?=w1617:bool)
    n603 = local read "stop"() -> (w1613:bool)
    n604 = And(x=w1617, y=w1615) -> (x .and. y?=→"click 2":bool)
    n605 = node-c288() -> ()  [unwired: 1 in, 1 out]
  }
  n606 = node-c288(w1) -> ()  [unwired: 1 out]
  n607 = property class="VI"(reference=w6, error in=w5, "Front Panel Window:Open"=TRUE) -> (reference out=w9:refnum<vi>, error out=w8:errorcluster)
  n608 = Close Reference(reference=w9, error in (no error)=w8) -> ()  [unwired: 1 out]
